vi "运维调试_氨氮.vi"() -> ()   [LabVIEW 2016, in "斯坦道氨氮.lvlib"]
uses:
  <vilib>/Utility/miscctls.llb/LVPointTypeDef.ctl
  <vilib>/Utility/config.llb/NI_LVConfig.lvlib
  <vilib>/ptbypt/NI_PtbyPt.lvlib
panel:
  out "模块版本号":string
  in  "校准按钮":T1
  out "单位:":T2(ring)
  out "运行状态":T3 {"数据时间:" format="%<%y/%m/%d %H:%M:%S>T"; "仪器时间:" format="%<%y/%m/%d %H:%M:%S>T"}
  out "二级权限":bool
  out "一级权限":bool
  out "输入密码":u32
  out "布尔":bool
  in  "仪器参数设置":bool
  in  "流程固件":bool
  in  "量程参数读取":T4
  in  "模块启用":bool
  in  "串口设置":bool
  in  "公式一键写入":bool
  in  "流程路径":path=path "C:/Users/STD/Documents/斯坦道流程文件/流程.xml"
  in  "曲线模型":cluster{"X^2":dbl, "X":dbl, "B":dbl, "r^2":dbl}(xcontrol)
  out "字符串":string
  in  "质控参数设置":bool
  in  "自动测试量程配置":T5
  out "温度2":sgl
  out "温度1":sgl
  out "ADC":sgl
  out "固件版本号":string
  in  "数组":string[](array[string])
  in  "量程切换阈值写入":bool
  in  "量程切换阈值读取":bool
  in  "参数下拉列表":enum16{"总磷", "总氮", "氨氮"}(ring)=enum."氨氮"
  in  "量程下拉列表":enum16{"低量程", "高量程"}(ring)
  in  "测量模式下拉列表":enum16{"水样测量", "零点核查", "跨度核查", "标样核查", "加标回收"}(ring)
  in  "公式":cluster{"X^2":dbl, "X":dbl, "b":dbl}
  in  "写公式":bool
  in  "读公式":bool
  in  "返回":bool
  in  "设置":bool
  out "集成报警信息":string
  out "定时启动":bool
  in  "停止":bool
  in  "手动启动":bool
  in  "单步测试":bool
  out "F3":sgl format="%#.6f"
  out "F2":sgl format="%#.6f"
  out "F1":sgl format="%#.6f"
  out "F0":sgl format="%#.6f"
  out "多列列表框":i32(listbox)
  # "参数设置"
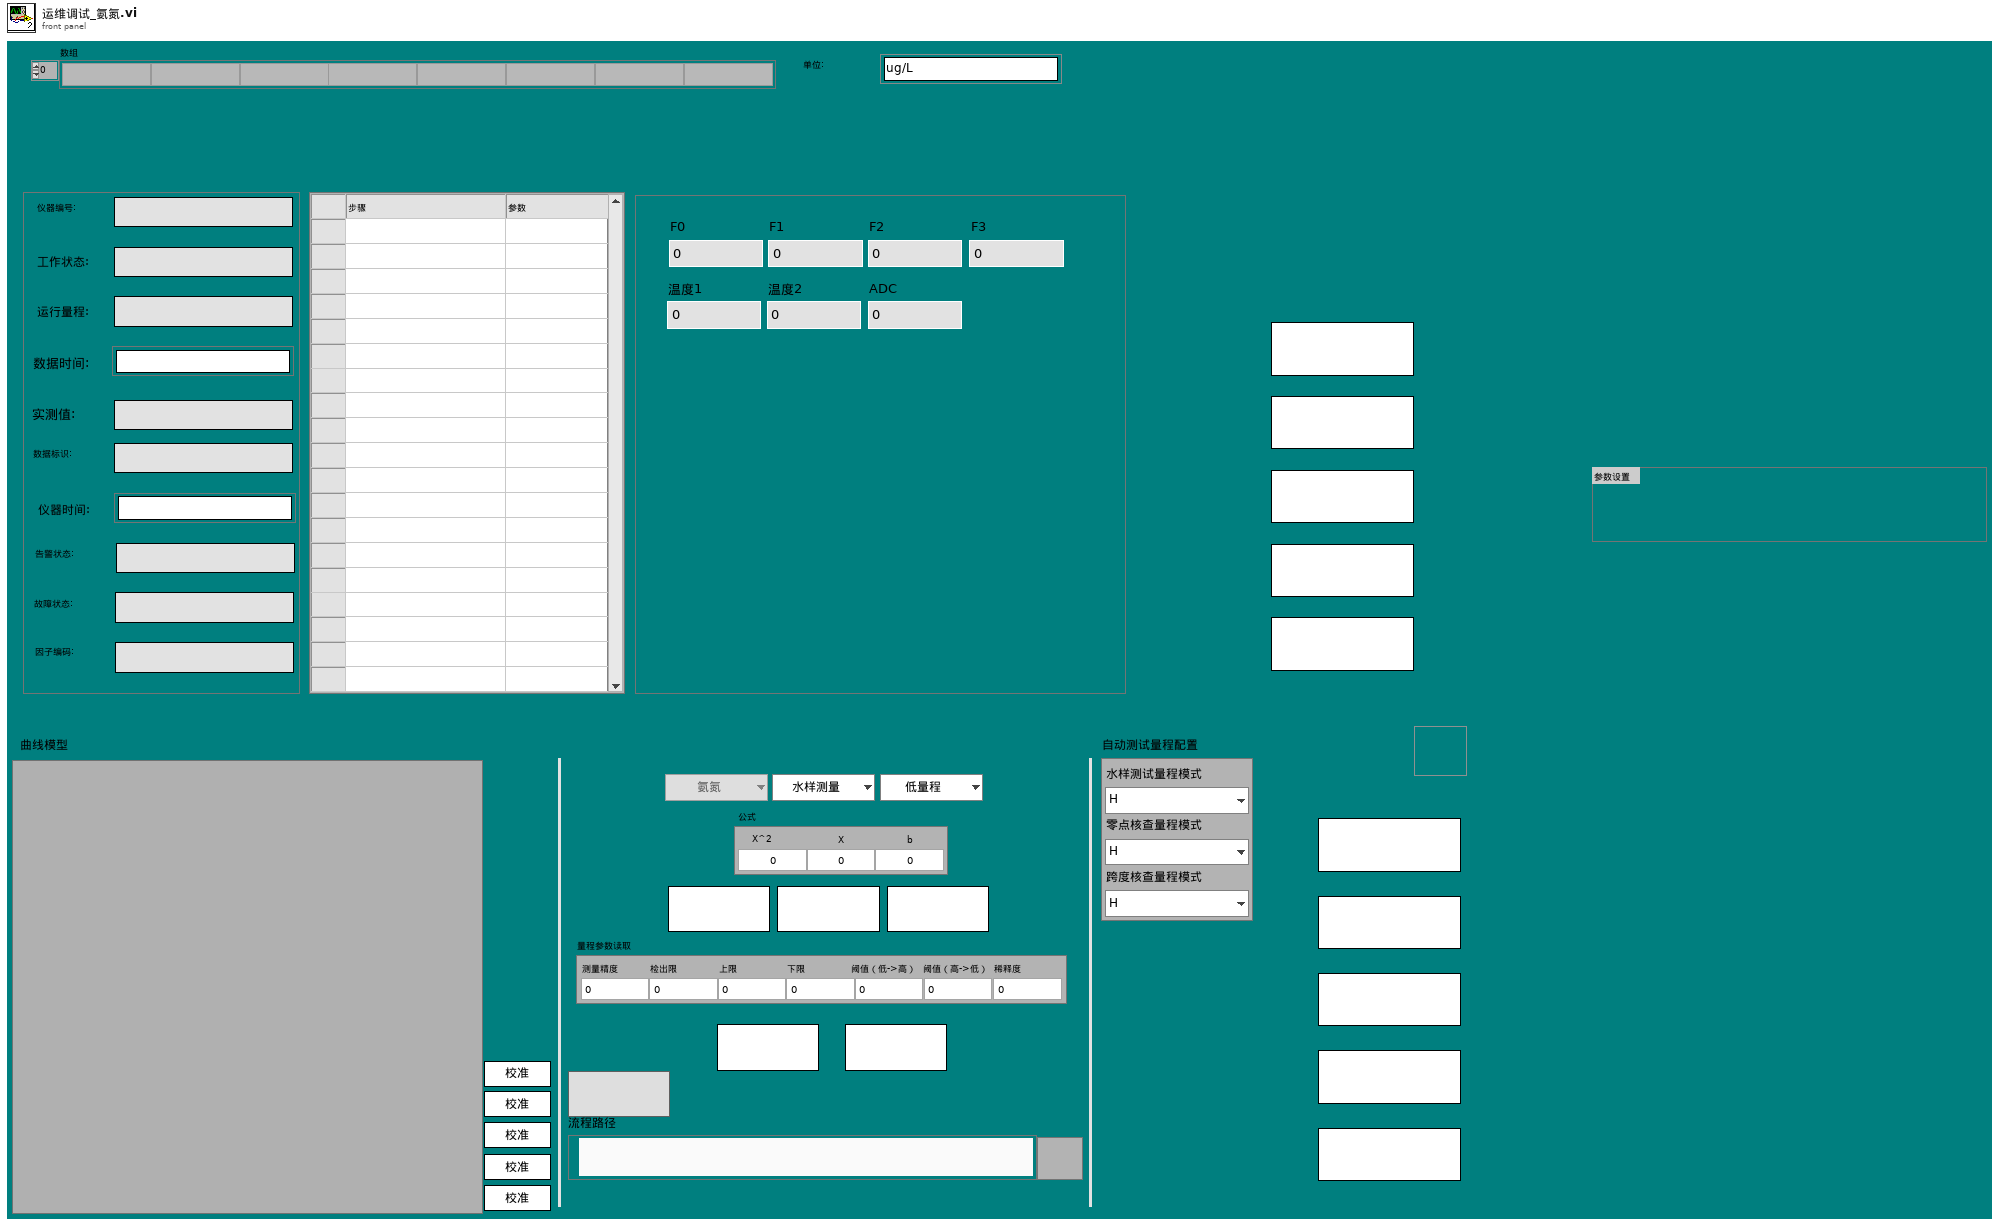
[diagram p1: front panel]
types:
  T1 = cluster{"校准1":bool, "校准2":bool, "校准3":bool, "校准4":bool, "校准5":bool}
  T2 = enum16{"ug/L", "mg/L", "ppm", "mg/m3", "cm", "ppb", "ug/m3", "%", "nmol/mol", "umol/mol", "MPN/L", "MPN/100ml", "ng/m3", "NTU", "无量纲", "ms/cm", "us/cm", "℃", "mV", "万个/L"}
  T3 = cluster{"仪器编号:":string, "工作状态:":string, "运行量程: ":string, "数据时间:":timestamp, "实测值:":string, "数据标识: ":string, "仪器时间:":timestamp, "告警状态: ":string, "故障状态:  ":string, "因子编码:":string}
  T4 = cluster{"测量精度":dbl, "检出限":dbl, "上限":dbl, "下限":dbl, "阈值（低->高）":dbl, "阈值（高->低）":dbl, "稀释度":dbl}
  T5 = cluster{"水样测试量程模式":enum16{"H", "L", "AUTO"}, "空白核查量程模式":enum16{"H", "L", "AUTO"}, "跨度核查量程模式":enum16{"H", "L", "AUTO"}}
  T6 = cluster{"Major":u16, "Minor":u16, "Fix":u16, "Build":u16}
  T7 = typedef "NI_LVConfig.lvlib/Config Data RefNum.ctl" = refnum<k1>
  T8 = enum16{"启动测量", "标样核查", "零点核查", "跨度核查", "空白测试", "平行样测试", "加标回收", "空白校准", "标样校准", "初始化（清洗）", "停止测试", "仪器重启", "校时", "模式设置", "测量间隔设置"}
  T9 = cluster{"控制命令":enum16{"启动测量", "标样核查", "零点核查", "跨度核查", "空白测试", "平行样测试", "加标回收", "空白校准", "标样校准", "初始化（清洗）", "停止测试", "仪器重启", "校时", "模式设置", "测量间隔设置"}, "周期设置类型":enum16{"定点启动", "间隔启动"}, "定时功能启用":bool, "定时间隔":dbl, "24H周期设置":bool[], "零点核查时间":u16, "跨度核查时间":u16, "质控频次":enum16{"关闭", "每天", "星期一", "星期二", "星期三", "星期四", "星期五", "星期六", "星期日"}}
  T10 = enum16{"关闭", "每天", "星期一", "星期二", "星期三", "星期四", "星期五", "星期六", "星期日"}
  T11 = typedef "LVDateTimeRec.ctl" = cluster{"秒数的小数部分":dbl, "秒":i32, "分":i32, "时":i32, "日":i32, "月":i32, "年":i32, "天数（周）":i32, "天数（年）":i32, "DST":i32}
  T12 = cluster{"系统时间":timestamp, "工作状态":enum16{"空闲", "水样测试", "标样核查", "零点核查", "跨度核查", "空白测试", "平行样测试", "加标回收", "空白校准", "标样校准", "初始化（清洗）"}, "测量模式":enum16{"待机", "连续模式", "周期模式", "定点模式", "受控模式", "手动模式"}, "告警代码":u16, "故障代码":u16, "日志代码":u16, "软件版本":u16, "F0":sgl, "F1":sgl, "F2":sgl, "F3":sgl, "T":sgl, "H":sgl, "id":u16, "flowid":u16, "量程":u16, "总磷控温温度1":sgl, "营养盐控温温度2":sgl, "ADC":sgl}
  T13 = enum16{"空闲", "水样测试", "标样核查", "零点核查", "跨度核查", "空白测试", "平行样测试", "加标回收", "空白校准", "标样校准", "初始化（清洗）"}
  T14 = enum32{"Bad", "Idle", "Run top level", "Running"}
  T15 = typedef "LVPointTypeDef.ctl" = cluster{"Horizontal":i16, "Vertical":i16}
  T16 = cluster{"因子编码":u32, "单位":u16, "标样参考值":sgl, "水样数据时间":timestamp, "水样实测值":sgl, "水样数据标识":string, "标样数据时间":timestamp, "标样实测值":sgl, "标样数据标识":string, "空白数据时间":timestamp, "空白实测值":sgl, "空白数据标识":string, "零点核查数据时间":timestamp, "零点核查实测值":sgl, "零点核查数据标识":string, "跨度核查数据时间":timestamp, "跨度核查实测值":sgl, "跨度核查数据标识":string, "加标回收数据时间":timestamp, "加标回收实测值":sgl, "加标回收数据标识":string, "平行样数据时间":timestamp, "平行样实测值":sgl, "平行样数据标识":string, "F0":sgl, "F1":sgl, "F2":sgl, "F3":sgl, "F4":sgl, "F5":sgl, "F6":sgl, "F7":sgl, "温度":sgl, "湿度":sgl, "X值":sgl, "fidrange":u16}
  T17 = enum8{"Enabled", "Disabled", "Disabled and Grayed Out"}
  T18 = cluster{"启动模式":enum16{"跨度核查", "水样测量", "空白核查", "标样核查", "加标回收"}, "启动参数":u16, "量程":enum16{"低量程", "高量程"}}
  T19 = cluster{"时间标识":timestamp, "设备":string, "日志信息":string, "流程参数":string}
  T20 = cluster{"时间标识":timestamp, "设备":string, "日志信息":string}
  T21 = typedef "LVRowAndColumnUnsignedTypeDef.ctl" = cluster{"Row":u32, "Column":u32}
  T22 = cluster{"参数下拉列表":enum16{"总磷", "总氮", "氨氮"}, "测量模式下拉列表":enum16{"水样测量", "零点核查", "跨度核查", "标样核查", "加标回收"}, "量程下拉列表":enum16{"低量程", "高量程"}}
  T23 = cluster{"站号":u16, "量程切换":enum32{"H", "L", "AUTO"}, "控制命令":enum16{"启动测量", "标样核查", "零点核查", "跨度核查", "空白测试", "平行样测试", "加标回收", "空白校准", "标样校准", "初始化（清洗）", "停止测试", "仪器重启", "校时", "模式设置", "测量间隔设置"}, "模式设置":enum16{"待机", "连续模式", "周期模式", "定点模式", "受控模式", "手动模式"}, "测量间隔":u16}
  T24 = cluster{"测量量程":dbl, "测量精度":dbl, "测量间隔":dbl, "消解温度":dbl, "消解时长":dbl, "空白校准时间":timestamp, "曲线截距":dbl, "曲线斜率":dbl, "测量检出限":dbl, "测量信号值":dbl, "线性相关系数":dbl, "二次多项式系数":dbl, "标样校准时间":timestamp, "单位":u16}
  T25 = cluster{"标液浓度1":dbl, "标液浓度2":dbl, "标液浓度3":dbl, "标液浓度4":dbl, "标液浓度5":dbl}
  T26 = cluster{"跨度值":dbl, "零点标准液浓度":dbl, "跨度标准液浓度":dbl, "标准液标准浓度":dbl}
  T27 = cluster{"确定":bool, "跨度值":dbl, "零点标准液浓度":dbl, "跨度标准液浓度":dbl, "标准液标准浓度":dbl}
  T28 = cluster{"确定":bool, "测量量程":dbl, "测量精度":dbl, "测量间隔":dbl, "消解温度":dbl, "消解时长":dbl, "空白校准时间":timestamp, "曲线截距":dbl, "曲线斜率":dbl, "测量检出限":dbl, "测量信号值":dbl, "线性相关系数":dbl, "二次多项式系数":dbl, "标样校准时间":timestamp, "单位":u16}
  T29 = cluster{"控制命令":enum16{"启动测量", "标样核查", "零点核查", "跨度核查", "空白测试", "平行样测试", "加标回收", "空白校准", "标样校准", "初始化（清洗）", "停止测试", "仪器重启", "校时", "模式设置", "测量间隔设置"}, "周期设置类型":enum16{"定点启动", "间隔启动"}, "定时功能启用":bool, "定时间隔":dbl, "24H周期设置":bool[], "空白核查时间":u16, "跨度核查时间":u16, "质控频次":enum16{"关闭", "每天", "星期一", "星期二", "星期三", "星期四", "星期五", "星期六", "星期日"}}
  T30 = cluster{"测量精度":u16, "检出限":dbl, "上限":dbl, "下限":dbl, "阈值（低->高）":dbl, "阈值（高->低）":dbl, "稀释度":dbl}
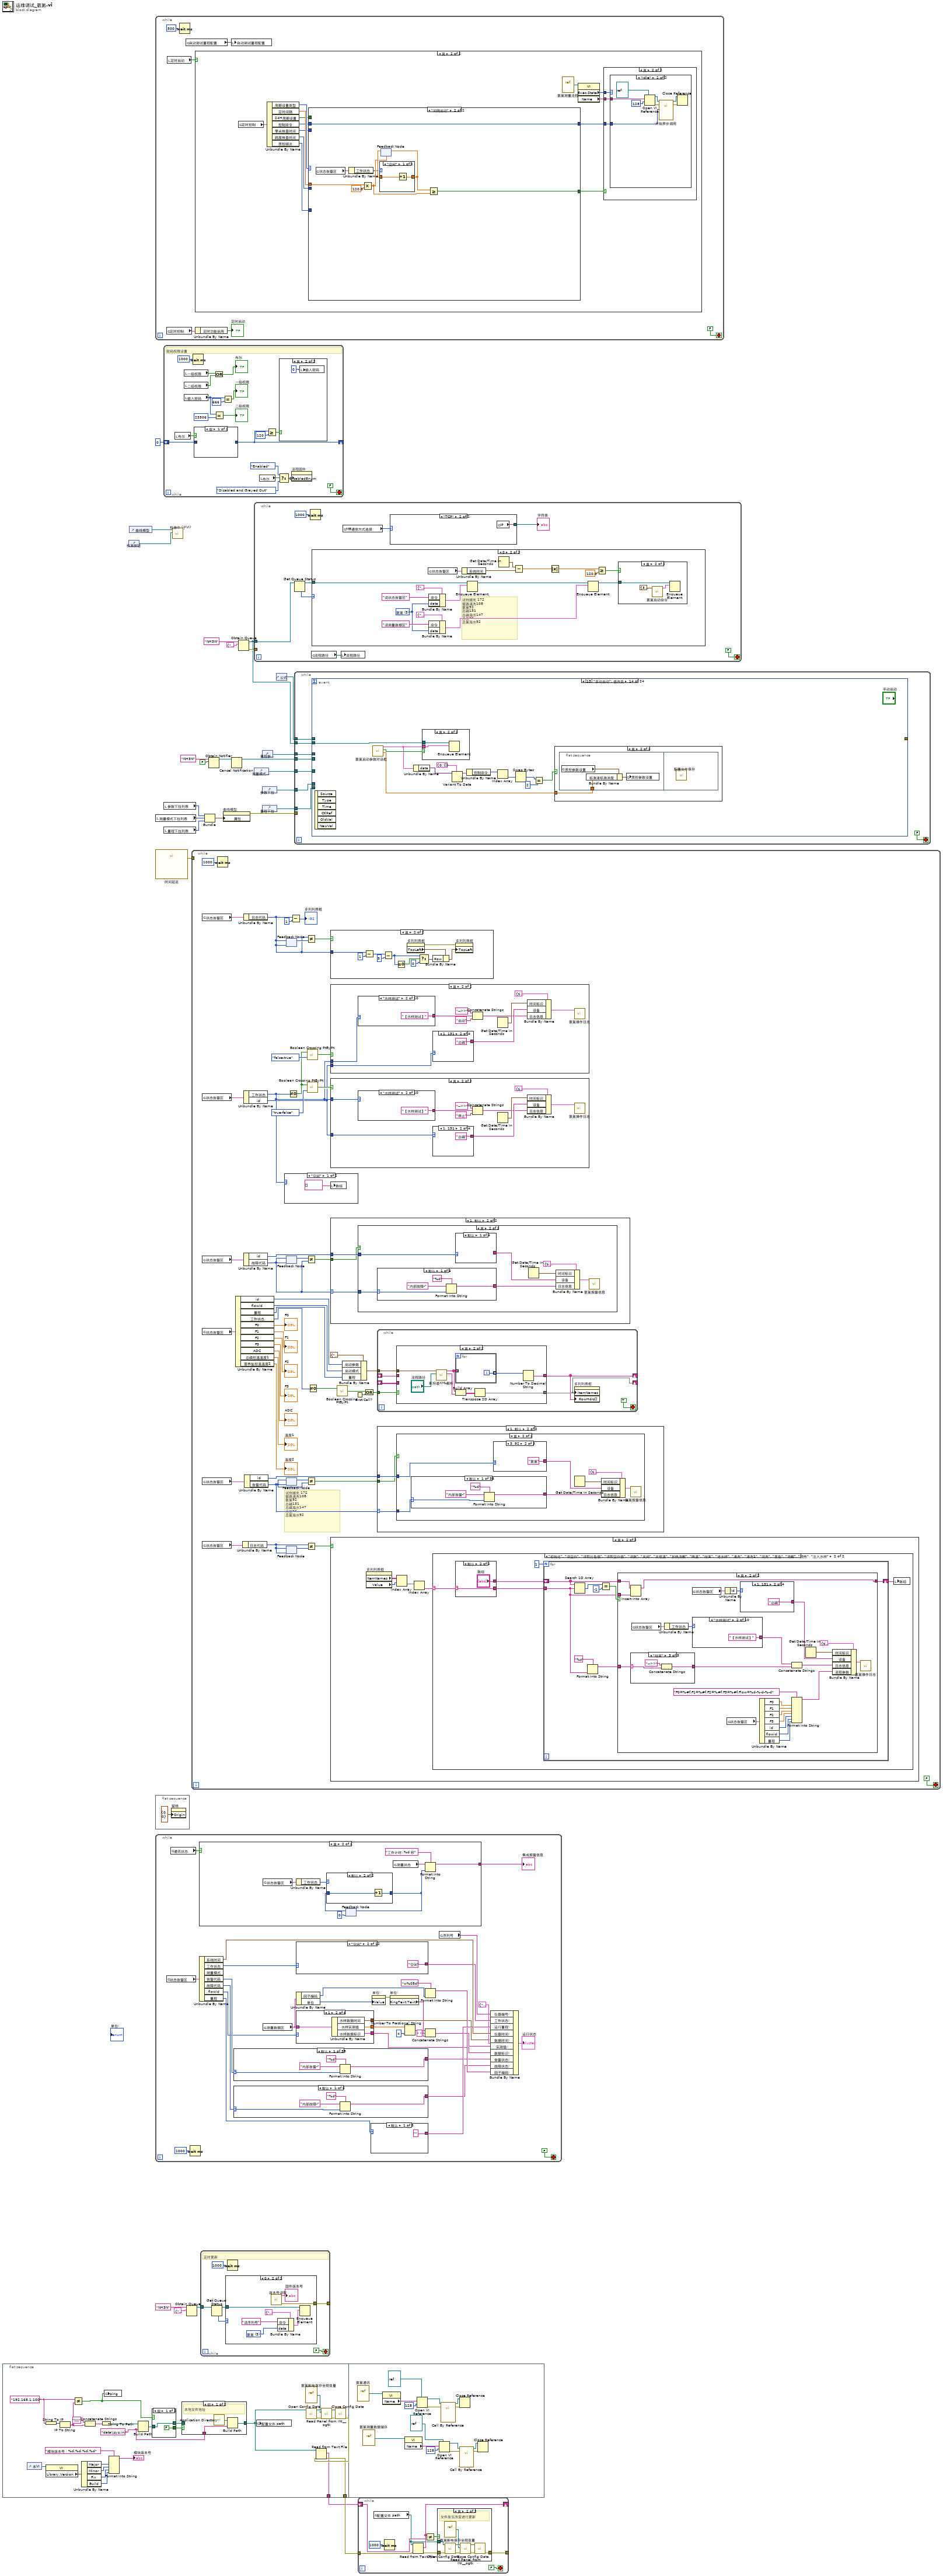
[diagram p0: block diagram]
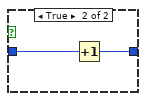
[diagram p4: hidden frame]
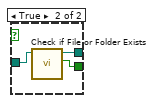
[diagram p5: hidden frame]
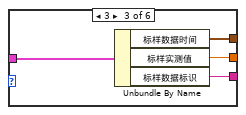
[diagram p9: hidden frame]
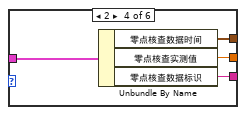
[diagram p10: hidden frame]
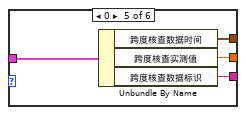
[diagram p11: hidden frame]
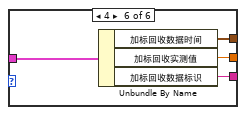
[diagram p12: hidden frame]
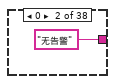
[diagram p13: hidden frame]
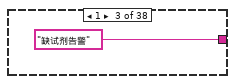
[diagram p14: hidden frame]
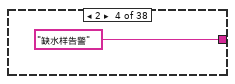
[diagram p15: hidden frame]
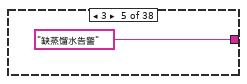
[diagram p16: hidden frame]
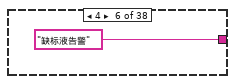
[diagram p17: hidden frame]
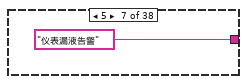
[diagram p18: hidden frame]
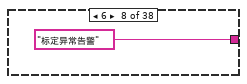
[diagram p19: hidden frame]
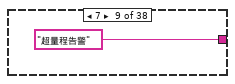
[diagram p20: hidden frame]
diagram:
  n1 = flat-sequence {
    tunnel: [w37] -> w4
    tunnel: [w36] -> w3
    frame #0 {
      w49 = "data\\sys.ini" ("名称或相对路径")
      w41 = "192.168.1.100" ("名称")
      n2 = control-ref of="本VI"() -> (w35:refnum<vi>)
      n3 = String To IP(1:w41) -> (0:w48:u32)
      n4 = property class="VI"(reference=w35) -> ("Library.Version"=w34:T6)  [unwired: 1 in, 2 out]
      n5 = IP To String(2:w48) -> (0:w45:string)  [unwired: 1 in]
      n6 = Not Equal?(x=w41, y=w45) -> (x != y?=w50:bool)
      n7 = Unbundle By Name(w34) -> ("Major"=w32:u16, "Minor"=w31:u16, "Fix"=w30:u16, "Build"=w29:u16)
      n8 = Concatenate Strings("\\\\" ("字符串"), w45) -> (w46:string)
      n9 = String To Path(string=w46) -> (path=w40:path)
      n10 = global write "VAR氨氮全局变量.vi" "ping"(w50) -> ()
      n11 = Format Into String(format string="模块版本号：%d.%d.%d.%d" ("格式字符串"), w32, w31, w30, w29) -> (resulting string=→"模块版本号":string)  [unwired: 2 in, 1 out]
      n12 = Build Path(base path=w40, name or relative path=w49) -> (appended path=w44:path)
      n13 = case shown="假" w50 {
        tunnel: w44 -> [w56 w60]
        tunnel: [w56 w59] -> w43
        tunnel: [FALSE w58] -> w42
        frame False {
        }
        frame True {
          n14 = call <vilib>:"Check if File or Folder Exists.vi"("path"=w60) -> ("file or folder exists?"=w58:bool, "dup path"=w59:path)  [unwired: 8 in, 1 out]
        }
      }
      n15 = case shown="假" w42 {
        tunnel: w43 -> [_ w64]
        tunnel: [w62 w64] -> w39
        tunnel: w49 -> [w61 _]
        frame False {
          # "本地文件地址"
          n16 = call <vilib>:"Application Directory.vi"() -> ("Application Directory"=w63:path)
          n17 = Build Path(base path=w63, name or relative path=w61) -> (appended path=w62:path)
        }
        frame True {
          # "网络共享地址"
        }
      }
      n18 = global write "VAR氨氮全局变量.vi" "配置文件 path"(w39) -> ()
      n19 = vi-ref "氨氮断电保存全局变量.vi"() -> (w54:refnum<vi>)
      n20 = call <vilib>:"Open Config Data.vi"("configuration file path"=w39) -> ("error out"=w52:errorcluster, "refnum"=w55:T7)  [unwired: 8 in, 1 out]
      n21 = call <userlib>:"Read Panel from INI__ogtk.vi"("error in (no error)"=w52, "VI ref"=w54, "refnum"=w55) -> ("error out"=w51:errorcluster, "refnum out"=w53:T7)  [unwired: 7 in]
      n22 = call <vilib>:"Close Config Data.vi"("error in (no error)"=w51, "refnum"=w53) -> ("error out"=w38:errorcluster)  [unwired: 8 in, 1 out]
      n23 = Read from Text File(file (use dialog)=w39, error in=w38) -> (text=w36:string, error out=w37:errorcluster)  [unwired: 2 in, 2 out]
    }
    frame #1 {
      n24 = vi-ref "氨氮通讯.vi"() -> (w80:refnum<vi>)
      n25 = vi-ref "氨氮测量数据储存.vi"() -> (w72:refnum<vi>)
      n26 = property class="VI"(reference=w80) -> ("Name"=w79:string)  [unwired: 1 in, 2 out]
      n27 = property class="VI"(reference=w72) -> ("Name"=w65:string)  [unwired: 1 in, 2 out]
      n28 = Open VI Reference(type specifier VI Refnum (for type only)=refnum<vi> refnum, vi path=w79, options=128 ("选项")) -> (vi reference=w77:refnum<vi>, error out=w75:errorcluster)  [unwired: 3 in]
      n29 = Open VI Reference(type specifier VI Refnum (for type only)=refnum<vi> refnum, vi path=w65, options=128 ("选项")) -> (vi reference=w67:refnum<vi>, error out=w69:errorcluster)  [unwired: 3 in]
      n30 = call-by-ref "?"(reference=w77, error in=w75) -> (reference out=w73:refnum<vi>, error out=w74:errorcluster)  [unwired: 12 in]
      n31 = Close Reference(reference=w73, error in (no error)=w74) -> ()  [unwired: 1 out]
      n32 = call-by-ref "?"(reference=w67, error in=w69) -> (reference out=w71:refnum<vi>, error out=w70:errorcluster)  [unwired: 12 in]
      n33 = Close Reference(reference=w71, error in (no error)=w70) -> ()  [unwired: 1 out]
    }
  }
  n34 = control-ref of="校准按钮"() -> (w1:refnum<vi>)
  n35 = control-ref of="曲线模型"() -> (w2:refnum<vi>)
  n36 = while {
    stop <- FALSE stop-if-true
    n37 = global read "氨氮断电保存全局变量.vi" "定时控制"() -> (w82:T9)
    n38 = local read "定时启动"() -> (w84:bool)
    n39 = Wait (ms)(milliseconds to wait=u32 500 ("等待时间（毫秒）")) -> ()  [unwired: 1 out]
    n40 = global read "氨氮断电保存全局变量.vi" "自动测试量程配置"() -> (w83:T5)
    n41 = case shown="真" w84 {
      frame False {
      }
      frame True {
        n42 = global read "氨氮断电保存全局变量.vi" "定时控制"() -> (w99:T9)
        n43 = Unbundle By Name(w99) -> ("周期设置类型"=w96:enum16{"定点启动", "间隔启动"}, "定时间隔"=w94:dbl, "24H周期设置"=w93:bool[], "控制命令"=w91:T8, "零点核查时间"=w90:u16, "跨度核查时间"=w89:u16, "质控频次"=w88:T10)
        n44 = case shown="\"间隔启动\"" w96 {
          tunnel: w94 -> [_ w157]
          tunnel: w93 -> [w123 _]
          tunnel: [w101 w155] -> w87
          tunnel: w91 -> [_ w153]
          tunnel: [w127 w153] -> w92
          tunnel: w88 -> [w126 _]
          tunnel: w90 -> [w119 _]
          tunnel: w89 -> [w108 _]
          frame "定点启动", Default {
            n45 = Get Date/Time In Seconds() -> (seconds since 1Jan1904=w125:timestamp)
            n46 = case shown="\"星期一\"..\"星期日\"" w126 {
              selector: w126 -> [_ _ w137]
              tunnel: w125 -> [_ _ w138]
              tunnel: [_ TRUE w134] -> w107
              frame "关闭", Default {
              }
              frame "每天" {
              }
              frame "星期一".."星期日" {
                n47 = case shown="\"星期日\"" w137 {
                  tunnel: ["" ("时间格式字符串(%c)") "星期一" ("时间格式字符串(%c)") "星期二" ("时间格式字符串(%c)") "星期三" ("时间格式字符串(%c)") "星期四" ("时间格式字符串(%c)") "星期五" ("时间格式字符串(%c)") "星期六" ("时间格式字符串(%c)") "星期日" ("时间格式字符串(%c)")] -> w136
                  frame "关闭", Default {
                  }
                  frame "星期一" {
                  }
                  frame "星期二" {
                  }
                  frame "星期三" {
                  }
                  frame "星期四" {
                  }
                  frame "星期五" {
                  }
                  frame "星期六" {
                  }
                  frame "星期日" {
                  }
                }
                n48 = Format Date/Time String(time format string (%c)="%A" ("时间格式字符串(%c)"), seconds (now)=w138) -> (date/time string=w135:string)  [unwired: 1 in]
                n49 = Equal?(x=w136, y=w135) -> (x = y?=w134:bool)
              }
            }
            n50 = Seconds To Date/Time(time stamp (now)=w125) -> (date time rec=w109:T11)  [unwired: 1 in]
            n51 = Unbundle By Name(w109) -> ("时"=w132:i32, "分"=w130:i32, "秒"=w131:i32)
            n52 = Unbundle By Name(w109) -> ("时"=w120:i32, "分"=w122:i32, "秒"=w121:i32)
            n53 = Unbundle By Name(w109) -> ("时"=w112:i32, "分"=w110:i32, "秒"=w111:i32)
            n54 = Equal?(x=w119, y=w120) -> (x = y?=w118:bool)
            n55 = Equal?(x=w108, y=w112) -> (x = y?=w113:bool)
            n56 = Equal To 0?(x=w130) -> (x = 0?=w129:bool)
            n57 = Equal To 0?(x=w131) -> (x = 0?=w128:bool)
            n58 = Equal To 0?(x=w122) -> (x = 0?=w117:bool)
            n59 = Equal To 0?(x=w121) -> (x = 0?=w116:bool)
            n60 = Equal To 0?(x=w110) -> (x = 0?=w114:bool)
            n61 = Equal To 0?(x=w111) -> (x = 0?=w115:bool)
            n62 = Index Array(array=w123, index=w132) -> (element=w124:bool)
            n63 = Compound Arithmetic op=AND ("复合运算")(w124, w129, w128) -> (w105:bool)
            n64 = Compound Arithmetic op=AND ("复合运算")(w107, w118, w117, w116) -> (w104:bool)
            n65 = Compound Arithmetic op=AND ("复合运算")(w107, w113, w114, w115) -> (w103:bool)
            n66 = Insert Into Array(array=bool[] [], new element #1=w105, new element #2=w104, new element #3=w103) -> (w102:bool[])  [unwired: 1 in]
            n67 = Boolean Array To Number(Boolean array=w102) -> (number=w100:u32)
            n68 = Not Equal To 0?(x=w100) -> (x != 0?=w101:bool)
            n69 = case shown="4" w100 {
              tunnel: [T8."启动测量" ("控制命令") T8."零点核查" ("控制命令") T8."跨度核查" ("控制命令")] -> w127
              frame 0, Default {
              }
              frame 2 {
              }
              frame 4 {
              }
            }
          }
          frame "间隔启动" {
            n70 = global read "VAR氨氮全局变量.vi" "状态告警区"() -> (w152:T12)
            n71 = Unbundle By Name(w152) -> ("工作状态"=w151:T13)
            n72 = Multiply(x=w157, y=120.0) -> (x*y=w154:dbl)
            n73 = feedback #1(w154) -> (w159:dbl)
            n74 = case shown="\"空闲\"" w151 {
              tunnel: w159 -> [w161 _]
              tunnel: [w160 _] -> w158
              frame "空闲" {
                n75 = Increment(x=w161) -> (x+1=w160:dbl)
              }
              frame "水样测试", Default {
              }
            }
            n76 = feedback-in #1(w158) -> ()
            n77 = Greater Or Equal?(x=w158, y=w154) -> (x >= y?=w155:bool)
          }
        }
        n78 = vi-ref "氨氮测量流程.vi"() -> (w98:refnum<vi>)
        n79 = property class="VI"(reference=w98) -> ("Exec.State"=w95:T14, "Name"=w97:string)  [unwired: 1 in, 2 out]
        n80 = case shown="真" w87 {
          tunnel: w97 -> [_ w164]
          tunnel: w92 -> [_ w163]
          tunnel: w95 -> [_ w162]
          frame False {
          }
          frame True {
            n81 = case shown="\"Idle\"" w162 {
              tunnel: w164 -> [_ w168]
              tunnel: w163 -> [_ w166]
              frame "Bad", Default {
              }
              frame "Idle" {
                n82 = Open VI Reference(type specifier VI Refnum (for type only)=refnum<vi> refnum, vi path=w168, options=128 ("选项")) -> (vi reference=w169:refnum<vi>, error out=w170:errorcluster)  [unwired: 3 in]
                n83 = call-by-ref "开始异步调用"(reference=w169, error in=w170, "控制命令"=w166) -> (reference out=w171:refnum<vi>, error out=w172:errorcluster)  [unwired: 11 in]
                n84 = Close Reference(reference=w171, error in (no error)=w172) -> ()  [unwired: 1 out]
              }
            }
          }
        }
      }
    }
    n85 = Unbundle By Name(w82) -> ("定时功能启用"=→"定时启动":bool)
    n86 = local write "自动测试量程配置"(w83) -> ()
  }
  n87 = local read "测量模式下拉列表"() -> (w7:enum16{"水样测量", "零点核查", "跨度核查", "标样核查", "加标回收"})
  n88 = call "时间延迟"() -> ("error out"=w19:errorcluster)  [unwired: 11 in]
  n89 = flat-sequence {
    frame #0 {
      n90 = property on="窗格" class="Pane"("Origin"=T15 {"Horizontal"=0, "Vertical"=0} ("原点")) -> ()  [unwired: 2 in, 2 out]
    }
  }
  n91 = while {
    stop <- FALSE stop-if-true
    n92 = global read "VAR氨氮全局变量.vi" "状态告警区"() -> (w201:T12)
    n93 = global read "VAR氨氮全局变量.vi" "通讯状态"() -> (w203:bool)
    n94 = Wait (ms)(milliseconds to wait=u32 1000 ("等待时间（毫秒）")) -> ()  [unwired: 1 out]
    n95 = case shown="真" w203 {
      tunnel: ["通讯异常" ("集成报警信息") w296] -> w202
      frame False {
      }
      frame True {
        n96 = global read "VAR氨氮全局变量.vi" "状态告警区"() -> (w302:T12)
        n97 = Unbundle By Name(w302) -> ("工作状态"=w301:T13)
        n98 = feedback #2(0) -> (w299:i32)
        n99 = case shown="默认" w301 {
          tunnel: w299 -> [_ w304]
          tunnel: [_ w303] -> w297
          frame "空闲" {
          }
          frame Default {
            n100 = Increment(x=w304) -> (x+1=w303:i32)
          }
        }
        n101 = feedback-in #2(w297) -> ()
        n102 = global read "VAR氨氮全局变量.vi" "测量状态"() -> (w295:string)
        n103 = Format Into String(format string="工作计时: %d 秒" ("格式字符串"), initial string=w295, w297) -> (resulting string=w296:string)  [unwired: 1 in, 1 out]
      }
    }
    "集成报警信息" <- w202
    n104 = Unbundle By Name(w201) -> ("系统时间"=w199:timestamp, "工作状态"=w190:T13, "告警代码"=w195:u16, "故障代码"=w194:u16, "flowid"=w189:u16, "量程"=w197:u16)  [unwired: 1 out]
    n105 = case shown="默认" w195 {
      selector: w195 -> [w227 _ _ _ _ _ _ _ _ _ _ _ _ _ _ _ _ _ _ _ _ _ _ _ _ _ _ _ _ _ _ _ _ _ _ _ _ _]
      tunnel: [w226 "无告警" "缺试剂告警" "缺水样告警" "缺蒸馏水告警" "缺标液告警" "仪表漏液告警" "标定异常告警" "超量程告警" "加热异常" "低试剂预警" "超上限告警" "超下限告警" "仪表内部其他异常" "滴定异常告警" "电极异常告警" "量程切换告警" "参数设置告警" "PH电极电位异常" "电导率电极异常" "浊度光度异常" "溶解氧电极异常" "溶解氧光强异常" "温度异常告警" "PH异常告警" "溶解氧异常告警" "电导率异常告警" "浊度异常告警" "叶绿素异常告警" "藻密度异常告警" "蓝绿藻异常告警" "ORP异常告警" "氨氮异常告警" "清洁刷异常告警" "SD卡异常告警" "蓝牙异常告警" "WiFi异常告警" "流程异常告警"] -> w178
      frame Default {
        n106 = Format Into String(format string="%d" ("格式字符串"), initial string="内部告警-" ("工作状态"), w227) -> (resulting string=w226:string)  [unwired: 1 in, 1 out]
      }
      frame 0 {
      }
      frame 1 {
      }
      frame 2 {
      }
      frame 3 {
      }
      frame 4 {
      }
      frame 5 {
      }
      frame 6 {
      }
      frame 7 {
      }
      frame 8 {
      }
      frame 9 {
      }
      frame 10 {
      }
      frame 11 {
      }
      frame 12 {
      }
      frame 13 {
      }
      frame 14 {
      }
      frame 15 {
      }
      frame 16 {
      }
      frame 17 {
      }
      frame 18 {
      }
      frame 19 {
      }
      frame 20 {
      }
      frame 21 {
      }
      frame 22 {
      }
      frame 23 {
      }
      frame 24 {
      }
      frame 25 {
      }
      frame 26 {
      }
      frame 27 {
      }
      frame 28 {
      }
      frame 29 {
      }
      frame 30 {
      }
      frame 31 {
      }
      frame 32 {
      }
      frame 33 {
      }
      frame 34 {
      }
      frame 35 {
      }
      frame 36 {
      }
    }
    n107 = case shown="默认" w194 {
      selector: w194 -> [w268 _ _ _ _ _]
      tunnel: [w267 "无故障" "电机故障" "温度故障" "通讯故障" "滴定故障"] -> w177
      frame Default {
        n108 = Format Into String(format string="%d" ("格式字符串"), initial string="内部故障-" ("工作状态"), w268) -> (resulting string=w267:string)  [unwired: 1 in, 1 out]
      }
      frame 0 {
      }
      frame 1 {
      }
      frame 2 {
      }
      frame 3 {
      }
      frame 4 {
      }
    }
    n109 = global read "VAR氨氮全局变量.vi" "测量数据区"() -> (w191:T16)
    n110 = case shown="\"空闲\"" w190 {
      selector: w190 -> [w279 _ _ _ _ _ _ _ _ _ _ _]
      tunnel: [w280 "空闲" ("工作状态") "水样测量" ("工作状态") "标样核查" ("工作状态") "零点核查" ("工作状态") "跨度核查" ("工作状态") "空白测试" ("工作状态") "平行样测试" ("工作状态") "加标回收" ("工作状态") "空白校准" ("工作状态") "标样校准" ("工作状态") "初始化" ("工作状态")] -> w198
      frame Default {
        n111 = Format Into String(format string="%d" ("格式字符串"), initial string="未知" ("工作状态"), w279) -> (resulting string=w280:string)  [unwired: 1 in, 1 out]
      }
      frame "空闲" {
      }
      frame "水样测试" {
      }
      frame "标样核查" {
      }
      frame "零点核查" {
      }
      frame "跨度核查" {
      }
      frame "空白测试" {
      }
      frame "平行样测试" {
      }
      frame "加标回收" {
      }
      frame "空白校准" {
      }
      frame "标样校准" {
      }
      frame "初始化（清洗）" {
      }
    }
    n112 = Unbundle By Name(w191) -> ("因子编码"=w192:u32, "单位"=w186:u16)
    n113 = case shown="1" w189 {
      tunnel: [_ w209 w213 w217 w221 w225] -> w180
      tunnel: [_ w207 w212 w216 w220 w224] -> w185
      tunnel: [_ w206 w211 w215 w219 w223] -> w179
      tunnel: w191 -> [_ w208 w210 w214 w218 w222]
      frame Default {
      }
      frame 1 {
        n114 = Unbundle By Name(w208) -> ("水样数据时间"=w209:timestamp, "水样实测值"=w207:sgl, "水样数据标识"=w206:string)
      }
      frame 3 {
        n115 = Unbundle By Name(w210) -> ("标样数据时间"=w213:timestamp, "标样实测值"=w212:sgl, "标样数据标识"=w211:string)
      }
      frame 2 {
        n116 = Unbundle By Name(w214) -> ("零点核查数据时间"=w217:timestamp, "零点核查实测值"=w216:sgl, "零点核查数据标识"=w215:string)
      }
      frame 0 {
        n117 = Unbundle By Name(w218) -> ("跨度核查数据时间"=w221:timestamp, "跨度核查实测值"=w220:sgl, "跨度核查数据标识"=w219:string)
      }
      frame 4 {
        n118 = Unbundle By Name(w222) -> ("加标回收数据时间"=w225:timestamp, "加标回收实测值"=w224:sgl, "加标回收数据标识"=w223:string)
      }
    }
    n119 = case shown="默认" w197 {
      tunnel: ["" ("字符串") "低量程" ("字符串") "高量程" ("字符串")] -> w196
      frame Default {
      }
      frame 0 {
      }
      frame 1 {
      }
    }
    n120 = property on="单位:" class="Enum (严格)"("Value"=w186) -> (error out=w187:errorcluster)  [unwired: 2 in, 1 out]
    n121 = property on="单位:" class="Enum (严格)"(error in=w187) -> ("RingText.Text"=w174:string)  [unwired: 1 in, 2 out]
    n122 = Number To Fractional String(number=w185, precision (6)=i16 4 ("精度(6)")) -> (F-format string=w183:string)  [unwired: 2 in]
    n123 = Format Into String(format string="w%05d" ("格式字符串"), w192) -> (resulting string=w181:string)  [unwired: 2 in, 1 out]
    n124 = Concatenate Strings(w183, " " ("字符串"), w174) -> (w182:string)
    n125 = global read "VAR氨氮全局变量.vi" "序列号"() -> (w200:string)
    n126 = Bundle By Name(cluster=T3 {"仪器编号:"="", "工作状态:"="", "运行量程: "="", "数据时间:"=timestamp(0 s since 1904-01-01), "实测值:"="", "数据标识: "="", "仪器时间:"=timestamp(0 s since 1904-01-01), "告警状态: "="", "故障状态:  "="", "因子编码:"=""} ("运行状态"), "仪器编号:"=w200, "工作状态:"=w198, "运行量程:"=w196, "仪器时间:"=w199, "数据时间:"=w180, "实测值:"=w182, "数据标识:"=w179, "告警状态:"=w178, "故障状态:"=w177, "因子编码:"=w181) -> (→"运行状态":T3)
  }
  n127 = while {
    shift-right: [w307] -> _
    shift-left: u32 0 ("等待时间（毫秒）") -> [w308]
    stop <- FALSE stop-if-true
    # "密码权限设置"
    n128 = local read "布尔"() -> (w309:bool)
    n129 = local read "一级权限"() -> (w316:bool)
    n130 = local read "二级权限"() -> (w317:bool)
    n131 = local read "输入密码"() -> (w320:u32)
    n132 = Wait (ms)(milliseconds to wait=u32 1000 ("等待时间（毫秒）")) -> ()  [unwired: 1 out]
    n133 = case shown="假" w309 {
      tunnel: w308 -> [_ w326]
      tunnel: [_ w325] -> w307
      frame False {
      }
      frame True {
        n134 = Increment(x=w326) -> (x+1=w325:u32)
      }
    }
    n135 = Or(x=w316, y=w317) -> (x .or. y?=→"布尔":bool)
    n136 = Equal?(x=w320, y=u32 23506) -> (x = y?=→"二级权限":bool)
    n137 = Equal?(x=w320, y=u32 666) -> (x = y?=→"一级权限":bool)
    n138 = local read "布尔"() -> (w311:bool)
    n139 = Greater Or Equal?(x=w307, y=u32 120) -> (x >= y?=w305:bool)
    n140 = Select(t=T17."Enabled" ("禁用"), s=w311, f=T17."Disabled and Grayed Out") -> (s? t:f=w312:T17)
    n141 = case shown="真" w305 {
      frame False {
      }
      frame True {
        n142 = local write "输入密码"(u32 0 ("输入密码")) -> ()
      }
    }
    n143 = property on="流程固件" class="Bool"("DisabledEnum"=w312) -> ()  [unwired: 2 in, 2 out]
  }
  n144 = local read "参数下拉列表"() -> (w8:enum16{"总磷", "总氮", "氨氮"})
  n145 = local read "量程下拉列表"() -> (w6:enum16{"低量程", "高量程"})
  n146 = call "校准中 (子VI).vi"("曲线模型"=w2, "校准按钮"=w1) -> ()  [unwired: 9 in]
  n147 = Obtain Queue(name (unnamed)="NH3N" ("名称（未命名）"), element data type=cluster{"命令":string, "data":variant} {"命令"="", "data"=variant}) -> (queue out=w16:refnum<queue>)  [unwired: 3 in, 2 out]
  n148 = while {
    tunnel: w19 -> [_]
    stop <- FALSE stop-if-true
    # "试剂填充 172 \n管路清洗108\n氨氮92\n总磷131\n总磷海水147\n总氮76\n总氮海水92"
    n149 = global read "VAR氨氮全局变量.vi" "状态告警区"() -> (w359:T12)
    n150 = global read "VAR氨氮全局变量.vi" "状态告警区"() -> (w347:T12)
    n151 = global read "VAR氨氮全局变量.vi" "状态告警区"() -> (w352:T12)
    n152 = global read "VAR氨氮全局变量.vi" "状态告警区"() -> (w367:T12)
    n153 = global read "VAR氨氮全局变量.vi" "状态告警区"() -> (w357:T12)
    n154 = global read "VAR氨氮全局变量.vi" "状态告警区"() -> (w345:T12)
    n155 = Wait (ms)(milliseconds to wait=u32 1000 ("等待时间（毫秒）")) -> ()  [unwired: 1 out]
    n156 = Unbundle By Name(w367) -> ("id"=w364:u16, "flowid"=w366:u16, "量程"=w365:u16, "工作状态"=w335:T13, "F0"=→"F0":sgl, "F1"=→"F1":sgl, "F2"=→"F2":sgl, "F3"=→"F3":sgl, "ADC"=→"ADC":sgl, "总磷控温温度1"=→"温度1":sgl, "营养盐控温温度2"=→"温度2":sgl)
    n157 = Unbundle By Name(w345) -> ("日志代码"=w344:u16)
    n158 = Unbundle By Name(w359) -> ("日志代码"=w341:u16)
    n159 = Unbundle By Name(w347) -> ("工作状态"=w328:T13, "id"=w327:u16)
    n160 = Unbundle By Name(w352) -> ("id"=w351:u16, "故障代码"=w348:u16)
    n161 = Unbundle By Name(w357) -> ("id"=w356:u16, "告警代码"=w353:u16)
    n162 = case shown="\"空闲\"" w328 {
      frame "空闲" {
        n163 = local write "数组"(string[] [] ("数组")) -> ()
      }
      frame "水样测试", Default {
      }
    }
    n164 = feedback-in #3(w341) -> ()
    n165 = feedback #3(w341) -> (w372:u16)
    n166 = feedback #4(w348) -> (w349:u16)
    n167 = feedback-in #4(w348) -> ()
    n168 = feedback #5(w353) -> (w354:u16)
    n169 = feedback-in #5(w353) -> ()
    n170 = feedback #6(w344) -> (w346:u16)
    n171 = feedback-in #6(w344) -> ()
    n172 = Not Equal To 0?(x=w328) -> (x != 0?=w330:bool)
    n173 = Subtract(x=w341, y=1) -> (x-y=→"多列列表框":i32)
    n174 = Not Equal?(x=w341, y=w372) -> (x != y?=w371:bool)
    n175 = Not Equal?(x=w349, y=w348) -> (x != y?=w350:bool)
    n176 = Not Equal?(x=w354, y=w353) -> (x != y?=w355:bool)
    n177 = Not Equal?(x=w344, y=w346) -> (x != y?=w343:bool)
    n178 = call <vilib>:"Boolean Crossing PtByPt.vi"("direction"=enum16{"either", "false-true", "true-false"}."false-true", "input"=w330) -> ("crossing"=w332:bool)  [unwired: 1 in]
    n179 = call <vilib>:"Boolean Crossing PtByPt.vi"("direction"=enum16{"either", "false-true", "true-false"}."true-false", "input"=w330) -> ("crossing"=w329:bool)  [unwired: 1 in]
    n180 = Not Equal To 0?(x=w335) -> (x != 0?=w369:bool)
    n181 = case shown="真" w371 {
      tunnel: w341 -> [_ w582]
      frame False {
      }
      frame True {
        n182 = Subtract(x=w582, y=1) -> (x-y=w580:i32)
        n183 = Subtract(x=w580, y=5) -> (x-y=w584:i32)
        n184 = Greater Or Equal To 0?(x=w584) -> (x >= 0?=w583:bool)
        n185 = property on="多列列表框" class="MCListbox (严格)"() -> (error out=w588:errorcluster, "TopLeft"=w589:T21)  [unwired: 2 in, 1 out]
        n186 = Select(t=w584, s=w583, f=0) -> (s? t:f=w585:i32)
        n187 = Bundle By Name(cluster=w589, "Row"=w585) -> (w590:T21)
        n188 = property on="多列列表框" class="MCListbox (严格)"(error in=w588, "TopLeft"=w590) -> ()  [unwired: 1 in, 2 out]
      }
    }
    n189 = case shown="真" w332 {
      tunnel: w327 -> [_ w402]
      tunnel: w328 -> [_ w401]
      frame False {
      }
      frame True {
        n190 = case shown="\"水样测试\"" w401 {
          tunnel: [_ "【水样测试】" ("字符串") "【标样核查】" ("字符串") "【零点核查】" ("字符串") "【跨度核查】" ("字符串") "【空白测试】" ("字符串") "【平行样测试】" ("字符串") "【加标回收】" ("字符串") "【空白校准】" ("字符串") "【标样校准】" ("字符串")] -> w400
          frame "空闲", Default {
          }
          frame "水样测试" {
          }
          frame "标样核查" {
          }
          frame "零点核查" {
          }
          frame "跨度核查" {
          }
          frame "空白测试" {
          }
          frame "平行样测试" {
          }
          frame "加标回收" {
          }
          frame "空白校准" {
          }
          frame "标样校准" {
          }
        }
        n191 = case shown="1, 131" w402 {
          tunnel: [_ "总磷" ("table输入") "氨氮" ("table输入") "总氮" ("table输入")] -> w404
          frame Default {
          }
          frame 1, 131 {
          }
          frame 3, 92 {
          }
          frame 2, 76 {
          }
        }
        n192 = Concatenate Strings("-->>" ("字符串"), w400, "启动" ("字符串")) -> (w399:string)
        n193 = Get Date/Time In Seconds() -> (seconds since 1Jan1904=w405:timestamp)
        n194 = Bundle By Name(cluster=T19 {"时间标识"=timestamp(0 s since 1904-01-01), "设备"="", "日志信息"="", "流程参数"=""} ("data in"), "时间标识"=w405, "设备"=w404, "日志信息"=w399) -> (w403:T19)
        n195 = call "氨氮操作日志.vi"("data in"=w403) -> ()  [unwired: 11 in]
      }
    }
    n196 = case shown="真" w329 {
      tunnel: w327 -> [_ w380]
      tunnel: w328 -> [_ w379]
      frame False {
      }
      frame True {
        n197 = case shown="\"水样测试\"" w379 {
          tunnel: [_ "【水样测试】" ("字符串") "【标样核查】" ("字符串") "【零点核查】" ("字符串") "【跨度核查】" ("字符串") "【空白测试】" ("字符串") "【平行样测试】" ("字符串") "【加标回收】" ("字符串") "【空白校准】" ("字符串") "【标样校准】" ("字符串")] -> w378
          frame "空闲", Default {
          }
          frame "水样测试" {
          }
          frame "标样核查" {
          }
          frame "零点核查" {
          }
          frame "跨度核查" {
          }
          frame "空白测试" {
          }
          frame "平行样测试" {
          }
          frame "加标回收" {
          }
          frame "空白校准" {
          }
          frame "标样校准" {
          }
        }
        n198 = case shown="1, 131" w380 {
          tunnel: [_ "总磷" ("table输入") "氨氮" ("table输入") "总氮" ("table输入")] -> w382
          frame Default {
          }
          frame 1, 131 {
          }
          frame 3, 92 {
          }
          frame 2, 76 {
          }
        }
        n199 = Concatenate Strings("-->>" ("字符串"), w378, "停止" ("字符串")) -> (w377:string)
        n200 = Get Date/Time In Seconds() -> (seconds since 1Jan1904=w383:timestamp)
        n201 = Bundle By Name(cluster=T19 {"时间标识"=timestamp(0 s since 1904-01-01), "设备"="", "日志信息"="", "流程参数"=""} ("data in"), "时间标识"=w383, "设备"=w382, "日志信息"=w377) -> (w381:T19)
        n202 = call "氨氮操作日志.vi"("data in"=w381) -> ()  [unwired: 11 in]
      }
    }
    n203 = case shown="1, 默认" w348 {
      selector: w348 -> [_ w487]
      tunnel: w351 -> [_ w488]
      tunnel: w350 -> [_ w486]
      frame 0 {
      }
      frame 1, Default {
        n204 = case shown="真" w486 {
          tunnel: w488 -> [_ w495]
          tunnel: w487 -> [_ w490]
          frame False {
          }
          frame True {
            n205 = case shown="默认" w490 {
              selector: w490 -> [w497 _ _ _ _ _]
              tunnel: [w496 "无故障" "电机故障" "温度故障" "通讯故障" "滴定故障"] -> w489
              frame Default {
                n206 = Format Into String(format string="%d" ("格式字符串"), initial string="内部故障-" ("工作状态"), w497) -> (resulting string=w496:string)  [unwired: 1 in, 1 out]
              }
              frame 0 {
              }
              frame 1 {
              }
              frame 2 {
              }
              frame 3 {
              }
              frame 4 {
              }
            }
            n207 = case shown="默认" w495 {
              tunnel: [_ "总磷" ("table输入") "氨氮" ("table输入") "总氮" ("table输入")] -> w491
              frame Default {
              }
              frame 1, 131 {
              }
              frame 3, 92 {
              }
              frame 2, 76 {
              }
            }
            n208 = Get Date/Time In Seconds() -> (seconds since 1Jan1904=w492:timestamp)
            n209 = Bundle By Name(cluster=T20 {"时间标识"=timestamp(0 s since 1904-01-01), "设备"="", "日志信息"=""} ("data in"), "时间标识"=w492, "设备"=w491, "日志信息"=w489) -> (w493:T20)
            n210 = call "氨氮报警信息.vi"("data in"=w493) -> ()  [unwired: 10 in, 1 out]
          }
        }
      }
    }
    n211 = case shown="真" w343 {
      frame False {
      }
      frame True {
        n212 = property on="多列列表框" class="MCListbox (严格)"() -> ("ItemNames"=w422:string[][], "Value"=w423:i32)  [unwired: 2 in, 2 out]
        n213 = Index Array(array=w422, index (row)=w423) -> (element=w421:string[])  [unwired: 1 in]
        n214 = Index Array(array=w421) -> (element=w420:string)  [unwired: 1 in]
        n215 = case shown="\"初始化\", \"读空白\", \"读取比色值\", \"读取空白值\", \"读数\", \"关阀\", \"关恒温\", \"加热消解\", \"降温\", \"结束\", \"进水样\", \"清洗\", \"清洗1\", \"润洗\", \"显色\", \"消解\", \"预热\", \"注入水样\"" w420 {
          selector: w420 -> [_ w426]
          frame Default {
          }
          frame "初始化", "读空白", "读取比色值", "读取空白值", "读数", "关阀", "关恒温", "加热消解", "降温", "结束", "进水样", "清洗", "清洗1", "润洗", "显色", "消解", "预热", "注入水样" {
            n216 = case shown="默认" w426 {
              selector: w426 -> [w430 w432]
              tunnel: [w430 w432] -> w425
              tunnel: [string[] [] ("数组") "数组"] -> w424
              frame "读数" {
              }
              frame Default {
              }
            }
            n217 = for {
              N: 1 -> [_]
              tunnel: w425 -> [w434]
              shift-right: [w433] -> w427
              shift-left: w424 -> [w435]
              n218 = Search 1D Array(1D array=w435, element=w434) -> (index of element=w438:i32)  [unwired: 1 in]
              n219 = Format Into String(format string="%s" ("格式字符串"), w434) -> (resulting string=w439:string)  [unwired: 2 in, 1 out]
              n220 = Equal?(x=w438, y=-1) -> (x = y?=w436:bool)
              n221 = case shown="真" w436 {
                tunnel: w439 -> [_ w447]
                tunnel: w435 -> [w441 w451]
                tunnel: w434 -> [_ w450]
                tunnel: [w441 w449] -> w433
                frame False {
                }
                frame True {
                  n222 = Insert Into Array(array=w451, new element=w450) -> (w449:string[])  [unwired: 1 in]
                  n223 = case shown="\"结束\"" w447 {
                    selector: w447 -> [w476 w479 w482]
                    tunnel: [w476 w478 w481] -> w443
                    frame Default {
                    }
                    frame "初始化" {
                      n224 = Concatenate Strings("-->>" ("字符串"), w479) -> (w478:string)
                    }
                    frame "结束" {
                      n225 = Concatenate Strings("-->>" ("字符串"), w482) -> (w481:string)
                    }
                  }
                  n226 = global read "VAR氨氮全局变量.vi" "状态告警区"() -> (w446:T12)
                  n227 = Unbundle By Name(w446) -> ("工作状态"=w445:T13)
                  n228 = global read "VAR氨氮全局变量.vi" "状态告警区"() -> (w466:T12)
                  n229 = case shown="\"水样测试\"" w445 {
                    tunnel: [_ "【水样测试】" ("字符串") "【标样核查】" ("字符串") "【零点核查】" ("字符串") "【跨度核查】" ("字符串") "【空白测试】" ("字符串") "【平行样测试】" ("字符串") "【加标回收】" ("字符串") "【空白校准】" ("字符串") "【标样校准】" ("字符串")] -> w444
                    frame "空闲", Default {
                    }
                    frame "水样测试" {
                    }
                    frame "标样核查" {
                    }
                    frame "零点核查" {
                    }
                    frame "跨度核查" {
                    }
                    frame "空白测试" {
                    }
                    frame "平行样测试" {
                    }
                    frame "加标回收" {
                    }
                    frame "空白校准" {
                    }
                    frame "标样校准" {
                    }
                  }
                  n230 = Unbundle By Name(w466) -> ("id"=w465:u16)
                  n231 = global read "VAR氨氮全局变量.vi" "状态告警区"() -> (w461:T12)
                  n232 = case shown="1, 131" w465 {
                    tunnel: [_ "总磷" ("table输入") "氨氮" ("table输入") "总氮" ("table输入")] -> w463
                    frame Default {
                    }
                    frame 1, 131 {
                    }
                    frame 3, 92 {
                    }
                    frame 2, 76 {
                    }
                  }
                  n233 = Unbundle By Name(w461) -> ("F0"=w458:sgl, "F1"=w457:sgl, "F2"=w456:sgl, "F3"=w455:sgl, "id"=w454:u16, "flowid"=w453:u16, "量程"=w452:u16)
                  n234 = Concatenate Strings(w444, w443) -> (w442:string)
                  n235 = Format Into String(format string="F0=%#f,F1=%#f,F2=%#f,F3=%#f,Flow=%d-%-d-%-d" ("格式字符串"), w458, w457, w456, w455, w454, w453, w452) -> (resulting string=w459:string)  [unwired: 2 in, 1 out]
                  n236 = Get Date/Time In Seconds() -> (seconds since 1Jan1904=w462:timestamp)
                  n237 = Bundle By Name(cluster=T19 {"时间标识"=timestamp(0 s since 1904-01-01), "设备"="", "日志信息"="", "流程参数"=""} ("data in"), "时间标识"=w462, "设备"=w463, "日志信息"=w442, "流程参数"=w459) -> (w464:T19)
                  n238 = call "氨氮操作日志.vi"("data in"=w464) -> ()  [unwired: 11 in]
                }
              }
            }
            n239 = local write "数组"(w427) -> ()
          }
        }
      }
    }
    n240 = call <vilib>:"Boolean Crossing PtByPt.vi"("input"=w369) -> ("crossing"=w334:bool)  [unwired: 2 in]
    n241 = Bundle By Name(cluster=T18 {"启动模式"=enum."跨度核查", "启动参数"=1, "量程"=enum."低量程"} ("参数簇"), "启动参数"=w364, "启动模式"=w366, "量程"=w365) -> (w358:T18)
    n242 = First Call?() -> (First Call?: T/F=w370:bool)
    n243 = Or(x=w334, y=w370) -> (x .or. y?=w368:bool)
    n244 = while {
      tunnel: w368 -> [w568]
      tunnel: w358 -> [w567]
      shift-right: [w562] -> _
      shift-left: _ -> [w564]
      shift-right: [w563] -> _
      shift-left: _ -> [w565]
      stop <- TRUE stop-if-true
      n245 = case shown="真" w568 {
        tunnel: [w570 w578] -> w563
        tunnel: [w569 w577] -> w562
        tunnel: w567 -> [_ w572]
        tunnel: w565 -> [w570 _]
        tunnel: w564 -> [w569 _]
        frame False {
        }
        frame True {
          n246 = call "斯坦道XML解析.vi"("添加的路径"="流程路径", "参数簇"=w572) -> ("步骤时间"=w573:string[], "步骤名"=w575:string[])  [unwired: 8 in]
          n247 = for {
            tunnel: w575 -> [_] mode=indexing
            tunnel: [w579] -> w576 mode=indexing
            i -> [w579]
          }
          n248 = Build Array(w575, w573) -> (w574:string[][])
          n249 = Transpose 2D Array(2D array=w574) -> (transposed array=w577:string[][])
          n250 = Number To Decimal String(number=w576) -> (decimal integer string=w578:string[])  [unwired: 1 in]
        }
      }
      n251 = property on="多列列表框" class="MCListbox (严格)"("ItemNames"=w562, "RowHdrs[]"=w563) -> ()  [unwired: 2 in, 2 out]
    }
    n252 = case shown="1, 默认" w353 {
      selector: w353 -> [_ w509]
      tunnel: w356 -> [_ w510]
      tunnel: w355 -> [_ w508]
      frame 0 {
      }
      frame 1, Default {
        n253 = case shown="真" w508 {
          tunnel: w510 -> [_ w517]
          tunnel: w509 -> [_ w511]
          frame False {
          }
          frame True {
            n254 = case shown="默认" w511 {
              selector: w511 -> [w519 _ _ _ _ _ _ _ _ _ _ _ _ _ _ _ _ _ _ _ _ _ _ _ _ _ _ _ _ _ _ _ _ _ _ _ _ _]
              tunnel: [w518 "无告警" "缺试剂告警" "缺水样告警" "缺蒸馏水告警" "缺标液告警" "仪表漏液告警" "标定异常告警" "超量程告警" "加热异常" "低试剂预警" "超上限告警" "超下限告警" "仪表内部其他异常" "滴定异常告警" "电极异常告警" "量程切换告警" "参数设置告警" "PH电极电位异常" "电导率电极异常" "浊度光度异常" "溶解氧电极异常" "溶解氧光强异常" "温度异常告警" "PH异常告警" "溶解氧异常告警" "电导率异常告警" "浊度异常告警" "叶绿素异常告警" "藻密度异常告警" "蓝绿藻异常告警" "ORP异常告警" "氨氮异常告警" "清洁刷异常告警" "SD卡异常告警" "蓝牙异常告警" "WiFi异常告警" "流程异常告警"] -> w512
              frame Default {
                n255 = Format Into String(format string="%d" ("格式字符串"), initial string="内部告警-" ("工作状态"), w519) -> (resulting string=w518:string)  [unwired: 1 in, 1 out]
              }
              frame 0 {
              }
              frame 1 {
              }
              frame 2 {
              }
              frame 3 {
              }
              frame 4 {
              }
              frame 5 {
              }
              frame 6 {
              }
              frame 7 {
              }
              frame 8 {
              }
              frame 9 {
              }
              frame 10 {
              }
              frame 11 {
              }
              frame 12 {
              }
              frame 13 {
              }
              frame 14 {
              }
              frame 15 {
              }
              frame 16 {
              }
              frame 17 {
              }
              frame 18 {
              }
              frame 19 {
              }
              frame 20 {
              }
              frame 21 {
              }
              frame 22 {
              }
              frame 23 {
              }
              frame 24 {
              }
              frame 25 {
              }
              frame 26 {
              }
              frame 27 {
              }
              frame 28 {
              }
              frame 29 {
              }
              frame 30 {
              }
              frame 31 {
              }
              frame 32 {
              }
              frame 33 {
              }
              frame 34 {
              }
              frame 35 {
              }
              frame 36 {
              }
            }
            n256 = case shown="3, 92" w517 {
              tunnel: ["总磷" ("table输入") "氨氮" ("table输入") "总氮" ("table输入")] -> w513
              frame 1, 131 {
              }
              frame 3, 92 {
              }
              frame 2, 76, Default {
              }
            }
            n257 = Get Date/Time In Seconds() -> (seconds since 1Jan1904=w514:timestamp)
            n258 = Bundle By Name(cluster=T20 {"时间标识"=timestamp(0 s since 1904-01-01), "设备"="", "日志信息"=""} ("data in"), "时间标识"=w514, "设备"=w513, "日志信息"=w512) -> (w515:T20)
            n259 = call "氨氮报警信息.vi"("data in"=w515) -> ()  [unwired: 10 in, 1 out]
          }
        }
      }
    }
  }
  n260 = while {
    tunnel: w16 -> [w595]
    tunnel: [w593] -> _
    stop <- FALSE stop-if-true
    # "定时更新"
    n261 = Get Queue Status(queue=w595) -> (queue out=w592:refnum<queue>, # elements in queue=w591:i32)  [unwired: 2 in, 6 out]
    n262 = case shown="0" w591 {
      tunnel: [_ w598] -> w593
      tunnel: w592 -> [_ w597]
      frame Default {
      }
      frame 0 {
        w601 = u16 3 items=["总磷"=1, "氨氮"=3] ("站号")
        n263 = call "版本号读取.vi"() -> ("error out"=w598:errorcluster, "固件版本号"=→"固件版本号":string)  [unwired: 10 in]
        n264 = Bundle By Name(cluster=cluster{"命令":string, "data":variant} {"命令"="", "data"=variant} ("元素"), "命令"="读序列号", "data"=w601) -> (w600:cluster{"命令":string, "data":variant})
        n265 = Enqueue Element(queue=w597, element=w600) -> ()  [unwired: 2 in, 3 out]
      }
    }
    n266 = Wait (ms)(milliseconds to wait=u32 1000 ("等待时间（毫秒）")) -> ()  [unwired: 1 out]
  }
  n267 = Bundle("参数下拉列表"=w8, "测量模式下拉列表"=w7, "量程下拉列表"=w6) -> (w9:T22)  [unwired: 1 in]
  n268 = Obtain Notifier(name (unnamed)="NH3N" ("名称（未命名）"), notification data type=FALSE) -> (notifier out=w12:refnum<notifier>)  [unwired: 2 in, 2 out]
  n269 = property on="曲线模型" class="曲线模型 (严格)"("属性"=w9) -> (error out=w15:errorcluster)  [unwired: 2 in, 1 out]
  n270 = Cancel Notification(0:w12) -> (8:w11:refnum<notifier>)  [unwired: 1 in, 2 out]
  n271 = Obtain Queue(name (unnamed)="NH3N" ("名称（未命名）"), element data type=cluster{"命令":string, "data":variant} {"命令"="", "data"=variant}) -> (queue out=w24:refnum<queue>, error out=w25:errorcluster)  [unwired: 3 in, 1 out]
  n272 = while {
    tunnel: w24 -> [w609]
    tunnel: w25 -> [_]
    stop <- FALSE stop-if-true
    n273 = Get Queue Status(queue=w609) -> (queue out=w605:refnum<queue>, # elements in queue=w604:i32)  [unwired: 2 in, 6 out]
    n274 = Wait (ms)(milliseconds to wait=u32 1000 ("等待时间（毫秒）")) -> ()  [unwired: 1 out]
    n275 = global read "氨氮断电保存全局变量.vi" "流程路径"() -> (w608:path)
    n276 = case shown="0" w604 {
      tunnel: w605 -> [_ w612]
      frame Default {
      }
      frame 0 {
        w621 = u16 3 items=["总磷"=1, "氨氮"=3] ("站号")
        # "试剂填充 172 \n管路清洗108\n氨氮92\n总磷131\n总磷海水147\n总氮76\n总氮海水92"
        n277 = global read "VAR氨氮全局变量.vi" "状态告警区"() -> (w613:T12)
        n278 = Bundle By Name(cluster=cluster{"命令":string, "data":variant} {"命令"="", "data"=variant} ("元素"), "命令"="读状态告警区", "data"=w621) -> (w627:cluster{"命令":string, "data":variant})
        n279 = Bundle By Name(cluster=cluster{"命令":string, "data":variant} {"命令"="", "data"=variant} ("元素"), "命令"="读测量数据区", "data"=w621) -> (w624:cluster{"命令":string, "data":variant})
        n280 = Unbundle By Name(w613) -> ("系统时间"=w620:timestamp)
        n281 = Enqueue Element(queue=w612, element=w627) -> (queue out=w622:refnum<queue>)  [unwired: 2 in, 2 out]
        n282 = Get Date/Time In Seconds() -> (seconds since 1Jan1904=w619:timestamp)
        n283 = Subtract(x=w619, y=w620) -> (x-y=w618:dbl)
        n284 = Absolute Value(x=w618) -> (abs(x)=w617:dbl)
        n285 = Enqueue Element(queue=w622, element=w624) -> (queue out=w614:refnum<queue>)  [unwired: 2 in, 2 out]
        n286 = Greater Or Equal?(x=w617, y=120.0) -> (x >= y?=w615:bool)
        n287 = case shown="真" w615 {
          tunnel: w614 -> [_ w630]
          frame False {
          }
          frame True {
            n288 = call "氨氮启动命令.vi"("参数"=T23 {"站号"=3, "量程切换"=enum."AUTO", "控制命令"=enum."校时", "模式设置"=enum."待机", "测量间隔"=0}) -> ("启动命令"=w629:cluster{"命令":string, "data":variant})  [unwired: 10 in]
            n289 = Enqueue Element(queue=w630, element=w629) -> ()  [unwired: 2 in, 3 out]
          }
        }
      }
    }
    n290 = local write "流程路径"(w608) -> ()
    n291 = global read "氨氮断电保存全局变量.vi" "MB通信方式选择"() -> (w606:enum16{"串口", "TCP"})
    n292 = case shown="\"TCP\"" w606 {
      tunnel: [w632 w633] -> w607
      frame "串口", Default {
        n293 = global read "氨氮断电保存全局变量.vi" "VISA Resource"() -> (w632:refnum<visa-resource-name>)
      }
      frame "TCP" {
        n294 = global read "氨氮断电保存全局变量.vi" "IP"() -> (w633:string)
      }
    }
    "字符串" <- w607
  }
  n295 = control-ref of="测量模式下拉列表"() -> (w21:refnum<vi>)
  n296 = control-ref of="量程参数读取"() -> (w10:refnum<vi>)
  n297 = control-ref of="参数下拉列表"() -> (w22:refnum<vi>)
  n298 = control-ref of="量程下拉列表"() -> (w23:refnum<vi>)
  n299 = control-ref of="公式"() -> (w20:refnum<vi>)
  n300 = while {
    tunnel: w24 -> [w640]
    tunnel: w23 -> [w639]
    tunnel: w22 -> [w638]
    tunnel: w21 -> [w637]
    tunnel: w20 -> [w636]
    tunnel: w10 -> [w635]
    tunnel: w15 -> [_]
    tunnel: w11 -> [w634]
    stop <- FALSE stop-if-true
    n301 = event shown="[13] \"手动启动\": 值改变" {
      selector: _ -> [_ _ _ _ _ _ _ _ _ _ _ _ _ _ _ _ _ _ _ _ _ _ _ _]
      dyn-events: _ -> [_ _ _ _ _ _ _ _ _ _ _ _ _ _ _ _ _ _ _ _ _ _ _ _]
      timeout: _ -> [_ _ _ _ _ _ _ _ _ _ _ _ _ _ _ _ _ _ _ _ _ _ _ _]
      tunnel: w640 -> [_ _ _ _ w660 w674 _ _ _ w694 _ _ _ w765 _ _ w780 _ _ _ _ _ _ _]
      tunnel: w639 -> [_ _ _ _ _ _ _ _ _ _ _ _ _ _ _ _ _ _ _ _ w796 _ _ _]
      tunnel: w638 -> [_ _ _ _ _ _ _ _ _ _ _ _ _ _ _ _ _ _ _ _ w794 _ w812 w819]
      tunnel: w637 -> [_ _ _ _ _ _ _ _ _ _ _ _ _ _ _ _ _ _ _ _ w795 _ _ _]
      tunnel: w636 -> [_ _ _ _ _ _ _ _ _ _ _ _ _ _ _ _ _ _ _ _ w790 _ _ _]
      tunnel: w635 -> [_ _ _ _ _ _ _ _ _ _ _ _ _ _ _ _ _ _ _ _ _ _ w810 _]
      tunnel: w634 -> [_ _ _ _ _ _ _ _ _ _ _ _ _ _ _ _ w775 _ _ _ _ _ _ _]
      tunnel: [_ _ _ w646 _ _ _ _ _ _ _ _ _ _ _ _ _ _ _ _ _ _ _ _] -> _
      event Timeout {
        n302 = event-data() -> ()  [unwired: 1 in, 3 out]
      }
      event "布尔": Mouse Down {
        n303 = event-data() -> ("CtlRef"=w643:refnum<vi>)  [unwired: 1 in, 5 out]
        n304 = property class="Bool (严格)"(reference=w643) -> ("Value"=w642:bool)  [unwired: 1 in, 2 out]
        n305 = case shown="真" w642 {
          frame False {
            n306 = call "密码键盘.vi"() -> ("NewNumber"=→"输入密码":dbl)  [unwired: 1 in]
          }
          frame True {
            n307 = local write "输入密码"(u32 0 ("输入密码")) -> ()
          }
        }
      }
      event "流程固件": Value Change {
        n308 = event-data() -> ()  [unwired: 1 in, 6 out]
        n309 = call "流程固件设置对话框.vi"() -> ()  [unwired: 12 in]
      }
      event "测量模式下拉列表", "量程下拉列表", "参数下拉列表": Value Change {
        n310 = event-data() -> ()  [unwired: 1 in, 6 out]
        n311 = local read "测量模式下拉列表"() -> (w649:enum16{"水样测量", "零点核查", "跨度核查", "标样核查", "加标回收"})
        n312 = local read "参数下拉列表"() -> (w648:enum16{"总磷", "总氮", "氨氮"})
        n313 = local read "量程下拉列表"() -> (w650:enum16{"低量程", "高量程"})
        n314 = Bundle("参数下拉列表"=w648, "测量模式下拉列表"=w649, "量程下拉列表"=w650) -> (w647:T22)  [unwired: 1 in]
        n315 = property on="曲线模型" class="曲线模型 (严格)"("属性"=w647) -> (error out=w646:errorcluster)  [unwired: 2 in, 1 out]
      }
      event "串口设置": Value Change {
        n316 = event-data() -> ()  [unwired: 1 in, 6 out]
        n317 = global read "氨氮断电保存全局变量.vi" "MB通信方式选择"() -> (w651:enum16{"串口", "TCP"})
        n318 = global read "氨氮断电保存全局变量.vi" "VISA Resource"() -> (w657:refnum<visa-resource-name>)
        n319 = global read "氨氮断电保存全局变量.vi" "PORT"() -> (w655:string)
        n320 = global read "氨氮断电保存全局变量.vi" "IP"() -> (w656:string)
        n321 = call "串口配置.vi"("PORT"=w655, "IP"=w656, "MB通信方式选择"=w651, "请选择串口:"=w657) -> ("PORT 2"=w653:string, "IP 2"=w654:string, "确认 2"=w658:bool, "VISA资源名称 2"=w659:refnum<visa-resource-name>, "MB通信方式选择 2"=w652:enum16{"串口", "TCP"})  [unwired: 3 in]
        n322 = case shown="真" w658 {
          tunnel: w659 -> [_ w665]
          tunnel: w660 -> [_ w664]
          tunnel: w654 -> [_ w663]
          tunnel: w653 -> [_ w662]
          tunnel: w652 -> [_ w661]
          frame False {
          }
          frame True {
            n323 = flat-sequence {
              tunnel: w665 -> [w670]
              tunnel: w664 -> [w671]
              tunnel: w663 -> [w669]
              tunnel: w662 -> [w668]
              tunnel: w661 -> [w667]
              frame #0 {
                n324 = global write "氨氮断电保存全局变量.vi" "IP"(w669) -> ()
                n325 = global write "氨氮断电保存全局变量.vi" "PORT"(w668) -> ()
                n326 = global write "氨氮断电保存全局变量.vi" "VISA Resource"(w670) -> ()
                n327 = global write "氨氮断电保存全局变量.vi" "MB通信方式选择"(w667) -> ()
                n328 = Flush Queue(queue=w671) -> (queue out=w666:refnum<queue>)  [unwired: 1 in, 2 out]
                n329 = Enqueue Element(queue=w666, element=cluster{"命令":string, "data":variant} {"命令"="启用模块", "data"=variant} ("元素")) -> ()  [unwired: 2 in, 3 out]
              }
              frame #1 {
                n330 = call "配置文件保存.vi"() -> ()  [unwired: 12 in]
              }
            }
          }
        }
      }
      event "模块启用": Value Change {
        n331 = event-data() -> ("OldVal"=w675:bool)  [unwired: 1 in, 5 out]
        n332 = Flush Queue(queue=w674) -> (queue out=w673:refnum<queue>)  [unwired: 1 in, 2 out]
        n333 = case shown="假" w675 {
          tunnel: w673 -> [w676 w678]
          frame False {
            n334 = Enqueue Element(queue=w676, element=cluster{"命令":string, "data":variant} {"命令"="停用模块", "data"=variant} ("元素")) -> ()  [unwired: 2 in, 3 out]
          }
          frame True {
            n335 = Enqueue Element(queue=w678, element=cluster{"命令":string, "data":variant} {"命令"="启用模块", "data"=variant} ("元素")) -> ()  [unwired: 2 in, 3 out]
          }
        }
      }
      event "流程路径": Value Change {
        n336 = event-data() -> ()  [unwired: 1 in, 6 out]
        n337 = flat-sequence {
          frame #0 {
            n338 = local read "流程路径"() -> (w680:path)
            n339 = global write "氨氮断电保存全局变量.vi" "流程路径"(w680) -> ()
          }
          frame #1 {
            n340 = call "配置文件保存.vi"() -> ()  [unwired: 12 in]
          }
        }
      }
      event "公式一键写入": Value Change {
        n341 = event-data() -> ()  [unwired: 1 in, 6 out]
        n342 = local read "公式"() -> (w681:cluster{"X^2":dbl, "X":dbl, "b":dbl})
        n343 = call "公式复合写入.vi"("公式"=w681) -> ()  [unwired: 11 in]
      }
      event "曲线模型": Value Change {
        n344 = event-data() -> ()  [unwired: 1 in, 6 out]
        n345 = Unbundle By Name("曲线模型") -> ("X^2"=w684:dbl, "X"=w685:dbl, "B"=w686:dbl, "r^2"=w687:dbl)
        n346 = Build Array(w684, w685, w686) -> (w683:dbl[])
        n347 = Array To Cluster(array=w683) -> (cluster=w682:cluster{"[0]":dbl, "[1]":dbl, "[2]":dbl})
        n348 = global read "氨氮断电保存全局变量.vi" "氨氮仪器参数"() -> (w690:T24)
        n349 = local write "公式"(w682) -> ()
        n350 = Bundle By Name(cluster=w690, "曲线截距"=w686, "曲线斜率"=w685, "线性相关系数"=w687, "二次多项式系数"=w684) -> (w689:T24)
        n351 = global write "氨氮断电保存全局变量.vi" "氨氮仪器参数"(w689) -> ()
      }
      event "校准按钮.校准1", "校准按钮.校准2", "校准按钮.校准3", "校准按钮.校准4", "校准按钮.校准5": Value Change {
        n352 = event-data() -> ("CtlRef"=w701:refnum<vi>)  [unwired: 1 in, 5 out]
        n353 = property on="曲线模型" class="曲线模型 (严格)"() -> ("浓度属性"=w697:T25)  [unwired: 2 in, 2 out]
        n354 = property class="Bool"(reference=w701) -> ("Label.Text"=w700:string)  [unwired: 1 in, 2 out]
        n355 = case shown="\"校准3\"" w700 {
          tunnel: [w704 w707 w710 w713 w716] -> w693
          tunnel: [u16 1 ("校准点1-5") u16 2 ("校准点1-5") u16 3 ("校准点1-5") u16 4 ("校准点1-5") u16 5 ("校准点1-5")] -> w698
          tunnel: w697 -> [w705 w708 w711 w714 w717]
          frame "校准1", Default {
            n356 = Unbundle By Name(w705) -> ("标液浓度1"=w704:dbl)
          }
          frame "校准2" {
            n357 = Unbundle By Name(w708) -> ("标液浓度2"=w707:dbl)
          }
          frame "校准3" {
            n358 = Unbundle By Name(w711) -> ("标液浓度3"=w710:dbl)
          }
          frame "校准4" {
            n359 = Unbundle By Name(w714) -> ("标液浓度4"=w713:dbl)
          }
          frame "校准5" {
            n360 = Unbundle By Name(w717) -> ("标液浓度5"=w716:dbl)
          }
        }
        n361 = Bundle By Name(cluster=cluster{"校准？":bool, "校准点1-5":u16, "校准浓度":dbl} {"校准？"=FALSE, "校准点1-5"=0, "校准浓度"=0.0} ("校准输出"), "校准？"=TRUE, "校准点1-5"=w698, "校准浓度"=w693) -> (w696:cluster{"校准？":bool, "校准点1-5":u16, "校准浓度":dbl})
        n362 = Not Equal To 0?(x=w693) -> (x != 0?=w692:bool)
        n363 = global write "氨氮断电保存全局变量.vi" "校准输出"(w696) -> ()
        n364 = case shown="真" w692 {
          tunnel: [cluster{"命令":string, "data":variant} {"命令"="启动", "data"=variant(cluster{"站号":u16, "控制命令":u16[]} {"站号"=3, "控制命令"=[2048, 0]})} ("启动命令") cluster{"命令":string, "data":variant} {"命令"="启动", "data"=variant(cluster{"站号":u16, "控制命令":u16[]} {"站号"=3, "控制命令"=[2304, 0]})} ("启动命令")] -> w691
          frame False {
            # "校零"
          }
          frame True {
            # "校标"
          }
        }
        n365 = Enqueue Element(queue=w694, element=w691) -> ()  [unwired: 2 in, 3 out]
      }
      event "质控参数设置": Value Change {
        n366 = event-data() -> ()  [unwired: 1 in, 6 out]
        n367 = global read "氨氮断电保存全局变量.vi" "质控参数设置"() -> (w719:T26)
        n368 = call "质控参数设置.vi"("质控参数设置"=w719) -> ("输出簇"=w720:T27)  [unwired: 10 in]
        n369 = Unbundle By Name(w720) -> ("确定"=w721:bool)
        n370 = case shown="真" w721 {
          tunnel: w720 -> [_ w723]
          tunnel: w719 -> [_ w722]
          frame False {
          }
          frame True {
            n371 = flat-sequence {
              tunnel: w723 -> [w730]
              tunnel: w722 -> [w729]
              frame #0 {
                n372 = Unbundle By Name(w730) -> ("跨度值"=w728:dbl, "零点标准液浓度"=w727:dbl, "跨度标准液浓度"=w726:dbl, "标准液标准浓度"=w725:dbl)
                n373 = Bundle By Name(cluster=w729, "跨度值"=w728, "零点标准液浓度"=w727, "跨度标准液浓度"=w726, "标准液标准浓度"=w725) -> (w724:T26)
                n374 = global write "氨氮断电保存全局变量.vi" "质控参数设置"(w724) -> ()
              }
              frame #1 {
                n375 = call "配置文件保存.vi"() -> ()  [unwired: 12 in]
              }
            }
          }
        }
      }
      event "仪器参数设置": Value Change {
        n376 = event-data() -> ()  [unwired: 1 in, 6 out]
        n377 = global read "氨氮断电保存全局变量.vi" "氨氮仪器参数"() -> (w731:T24)
        n378 = call "仪器参数设置.vi"("仪器参数设置"=w731) -> ("仪器参数设置输出"=w732:T28)  [unwired: 10 in]
        n379 = Unbundle By Name(w732) -> ("确定"=w733:bool)
        n380 = case shown="真" w733 {
          tunnel: w732 -> [_ w735]
          tunnel: w731 -> [_ w734]
          frame False {
          }
          frame True {
            n381 = flat-sequence {
              tunnel: w735 -> [w752]
              tunnel: w734 -> [w751]
              frame #0 {
                n382 = Unbundle By Name(w752) -> ("测量量程"=w750:dbl, "测量精度"=w749:dbl, "测量间隔"=w748:dbl, "消解温度"=w747:dbl, "消解时长"=w745:dbl, "空白校准时间"=w744:timestamp, "曲线截距"=w743:dbl, "曲线斜率"=w742:dbl, "测量检出限"=w741:dbl, "测量信号值"=w740:dbl, "线性相关系数"=w739:dbl, "二次多项式系数"=w738:dbl, "标样校准时间"=w737:timestamp, "单位"=w736:u16)
                n383 = Bundle By Name(cluster=w751, "测量量程"=w750, "测量精度"=w749, "测量间隔"=w748, "消解温度"=w747, "消解时长"=w745, "空白校准时间"=w744, "曲线截距"=w743, "曲线斜率"=w742, "测量检出限"=w741, "测量信号值"=w740, "线性相关系数"=w739, "二次多项式系数"=w738, "标样校准时间"=w737, "单位"=w736) -> (w746:T24)
                n384 = global write "氨氮断电保存全局变量.vi" "氨氮仪器参数"(w746) -> ()
              }
              frame #1 {
                n385 = call "配置文件保存.vi"() -> ()  [unwired: 12 in]
              }
            }
          }
        }
      }
      event "自动测试量程配置": Value Change {
        n386 = event-data() -> ()  [unwired: 1 in, 6 out]
        n387 = flat-sequence {
          frame #0 {
            n388 = global write "氨氮断电保存全局变量.vi" "自动测试量程配置"("自动测试量程配置") -> ()
          }
          frame #1 {
            n389 = call "配置文件保存.vi"() -> ()  [unwired: 12 in]
          }
        }
      }
      event "手动启动": Value Change {
        n390 = event-data() -> ()  [unwired: 1 in, 6 out]
        n391 = call "氨氮启动参数对话框.vi"() -> ("标样浓度输出"=w754:dbl, "确认"=w764:bool, "元素"=w763:cluster{"命令":string, "data":variant})  [unwired: 9 in]
        n392 = Unbundle By Name(w763) -> ("data"=w761:variant)
        n393 = case shown="真" w764 {
          tunnel: w765 -> [_ w771]
          tunnel: w763 -> [_ w770]
          frame False {
          }
          frame True {
            n394 = Enqueue Element(queue=w771, element=w770) -> ()  [unwired: 2 in, 3 out]
          }
        }
        n395 = Variant To Data(type=cluster{"站号":u16, "控制命令":u16[]} {"站号"=0, "控制命令"=[]} ("输出簇"), Variant=w761) -> (data=w760:cluster{"站号":u16, "控制命令":u16[]})  [unwired: 1 in, 1 out]
        n396 = Unbundle By Name(w760) -> ("控制命令"=w759:u16[])
        n397 = Index Array(array=w759) -> (element=w758:u16)  [unwired: 1 in]
        n398 = Swap Bytes(anything=w758) -> (byte swapped=w757:u16)
        n399 = Equal?(x=w757, y=u16 2) -> (x = y?=w755:bool)
        n400 = case shown="真" w755 {
          tunnel: w754 -> [_ w766]
          frame False {
          }
          frame True {
            n401 = flat-sequence {
              tunnel: w766 -> [w767]
              frame #0 {
                n402 = global read "氨氮断电保存全局变量.vi" "质控参数设置"() -> (w769:T26)
                n403 = Bundle By Name(cluster=w769, "标准液标准浓度"=w767) -> (w768:T26)
                n404 = global write "氨氮断电保存全局变量.vi" "质控参数设置"(w768) -> ()
              }
              frame #1 {
                n405 = call "配置文件保存.vi"() -> ()  [unwired: 12 in]
              }
            }
          }
        }
      }
      event "定时启动": Mouse Down {
        n406 = event-data() -> ()  [unwired: 1 in, 6 out]
        n407 = flat-sequence {
          frame #0 {
            n408 = global read "氨氮断电保存全局变量.vi" "定时控制"() -> (w773:T9)
            n409 = call "周期设置.vi"("定时控制输入"=w773) -> ("定时控制输出"=w772:T29)  [unwired: 10 in]
            n410 = global write "氨氮断电保存全局变量.vi" "定时控制"(w772) -> ()
          }
          frame #1 {
            n411 = call "配置文件保存.vi"() -> ()  [unwired: 12 in]
          }
        }
      }
      event "单步测试": Value Change {
        n412 = event-data() -> ()  [unwired: 1 in, 6 out]
        n413 = call "氨氮单步调试对话框.vi"() -> ()  [unwired: 12 in]
      }
      event "停止": Value Change {
        n414 = event-data() -> ()  [unwired: 1 in, 6 out]
        n415 = Enqueue Element(queue=w780, element=cluster{"命令":string, "data":variant} {"命令"="启动", "data"=variant(cluster{"站号":u16, "控制命令输出":u16[]} {"站号"=1, "控制命令输出"=[2816]})} ("元素")) -> (queue out=w777:refnum<queue>)  [unwired: 2 in, 2 out]
        n416 = Cancel Notification(0:w775) -> (8:w776:refnum<notifier>)  [unwired: 1 in, 2 out]
        n417 = Send Notification(notification=TRUE ("通知"), notifier=w776) -> ()  [unwired: 1 in, 2 out]
        n418 = Enqueue Element(queue=w777, element=cluster{"命令":string, "data":variant} {"命令"="启动", "data"=variant(cluster{"站号":u16, "控制命令输出":u16[]} {"站号"=2, "控制命令输出"=[2816]})} ("元素")) -> ()  [unwired: 2 in, 3 out]
      }
      event "设置": Value Change {
        n419 = event-data() -> ()  [unwired: 1 in, 6 out]
        n420 = property on="窗格" class="Pane"("Origin"=T15 {"Horizontal"=0, "Vertical"=628} ("原点")) -> ()  [unwired: 2 in, 2 out]
      }
      event "返回": Value Change {
        n421 = event-data() -> ()  [unwired: 1 in, 6 out]
        n422 = property on="窗格" class="Pane"("Origin"=T15 {"Horizontal"=0, "Vertical"=0} ("原点")) -> ()  [unwired: 2 in, 2 out]
      }
      event "公式.X^2", "公式.X", "公式.b": Mouse Down {
        n423 = event-data() -> ("CtlRef"=w786:refnum<vi>)  [unwired: 1 in, 5 out]
        n424 = property class="DigNum (严格)"(reference=w786) -> (reference out=w784:refnum<vi>, "Value"=w785:dbl)  [unwired: 1 in, 1 out]
        n425 = call "数字键盘.vi"("OldNumber"=w785) -> ("NewNumber"=w783:dbl)
        n426 = property class="DigNum (严格)"(reference=w784, "Val(Sgnl)"=w783) -> ()  [unwired: 1 in, 2 out]
      }
      event "读公式": Value Change {
        n427 = event-data() -> ()  [unwired: 1 in, 6 out]
        n428 = property class="Enum (严格)"(reference=w795) -> ("Value"=w792:enum16{"水样测量", "零点核查", "跨度核查", "标样核查", "加标回收"})  [unwired: 1 in, 2 out]
        n429 = property class="Enum (严格)"(reference=w794) -> ("Value"=w793:enum16{"总磷", "总氮", "氨氮"})  [unwired: 1 in, 2 out]
        n430 = property class="Enum (严格)"(reference=w796) -> ("Value"=w791:enum16{"低量程", "高量程"})  [unwired: 1 in, 2 out]
        n431 = call "公式读取.vi"("量程"=w791, "测量模式"=w792, "测量参数"=w793) -> ("error out"=w788:errorcluster, "公式"=w789:cluster{"X^2":dbl, "X":dbl, "b":dbl})  [unwired: 7 in]
        n432 = property class="Clust (严格)"(reference=w790, "Value"=w789) -> ()  [unwired: 1 in, 2 out]
        n433 = case shown="错误" w788 {
          tunnel: ["读取成功" ("消息") "读取失败" ("消息")] -> w787
          frame No Error {
          }
          frame Error {
          }
        }
        n434 = One Button Dialog(message=w787) -> ()  [unwired: 1 in, 1 out]
      }
      event "写公式": Value Change {
        n435 = event-data() -> ()  [unwired: 1 in, 6 out]
        n436 = call "公式写入.vi"("公式"="公式", "量程"="量程下拉列表", "测量模式"="测量模式下拉列表", "测量参数"="参数下拉列表") -> ("error out"=w801:errorcluster)  [unwired: 7 in]
        n437 = case shown="无错误" w801 {
          tunnel: ["写入成功" ("消息") "写入失败" ("消息")] -> w802
          frame No Error {
          }
          frame Error {
          }
        }
        n438 = One Button Dialog(message=w802) -> ()  [unwired: 1 in, 1 out]
      }
      event "量程切换阈值读取": Value Change {
        n439 = event-data() -> ()  [unwired: 1 in, 6 out]
        n440 = property class="Enum (严格)"(reference=w812) -> ("Value"=w811:enum16{"总磷", "总氮", "氨氮"})  [unwired: 1 in, 2 out]
        n441 = call "量程读取.vi"("测量参数"=w811) -> ("error out"=w807:errorcluster, "量程参数读取"=w809:T30)  [unwired: 9 in]
        n442 = property class="Clust (严格)"(reference=w810, "Value"=w809) -> ()  [unwired: 1 in, 2 out]
        n443 = case shown="错误" w807 {
          tunnel: ["读取成功" ("消息") "读取失败" ("消息")] -> w808
          frame No Error {
          }
          frame Error {
          }
        }
        n444 = One Button Dialog(message=w808) -> ()  [unwired: 1 in, 1 out]
      }
      event "量程切换阈值写入": Value Change {
        n445 = event-data() -> ()  [unwired: 1 in, 6 out]
        n446 = property class="Enum (严格)"(reference=w819) -> ("Value"=w818:enum16{"总磷", "总氮", "氨氮"})  [unwired: 1 in, 2 out]
        n447 = call "量程写入.vi"("量程参数写入"="量程参数读取", "测量参数"=w818) -> ("error out"=w816:errorcluster)  [unwired: 8 in]
        n448 = case shown="无错误" w816 {
          tunnel: ["写入成功" ("消息") "写入失败" ("消息")] -> w817
          frame No Error {
          }
          frame Error {
          }
        }
        n449 = One Button Dialog(message=w817) -> ()  [unwired: 1 in, 1 out]
      }
    }
  }
  n450 = while {
    tunnel: [w829] -> _
    shift-right: [w827] -> _
    shift-left: w3 -> [w826]
    tunnel: w4 -> [w823]
    stop <- FALSE stop-if-true
    n451 = global read "VAR氨氮全局变量.vi" "配置文件 path"() -> (w822:path)
    n452 = Wait (ms)(milliseconds to wait=u32 1000 ("等待时间（毫秒）")) -> ()  [unwired: 1 out]
    n453 = Read from Text File(file (use dialog)=w822, error in=w823) -> (text=w827:string, error out=w824:errorcluster)  [unwired: 2 in, 2 out]
    n454 = Not Equal?(x=w827, y=w826) -> (x != y?=w825:bool)
    n455 = case shown="真" w825 {
      tunnel: [w831 w835] -> w829
      tunnel: w822 -> [_ w834]
      tunnel: w824 -> [w831 w833]
      frame False {
      }
      frame True {
        # "文件发生改变进行更新"
        n456 = vi-ref "氨氮断电保存全局变量.vi"() -> (w832:refnum<vi>)
        n457 = call <vilib>:"Open Config Data.vi"("error in (no error)"=w833, "configuration file path"=w834) -> ("error out"=w839:errorcluster, "refnum"=w838:T7)  [unwired: 7 in, 1 out]
        n458 = call <userlib>:"Read Panel from INI__ogtk.vi"("error in (no error)"=w839, "VI ref"=w832, "refnum"=w838) -> ("error out"=w837:errorcluster, "refnum out"=w836:T7)  [unwired: 7 in]
        n459 = call <vilib>:"Close Config Data.vi"("error in (no error)"=w837, "refnum"=w836) -> ("error out"=w835:errorcluster)  [unwired: 8 in, 1 out]
      }
    }
  }
